vi "frontend3.vi"() -> ()   [LabVIEW 2011]
uses:
  custom_modules/typedefs/preset_control_cluster.ctl
  custom_modules/typedefs/control_cluster.ctl
  custom_modules/typedefs/origin_controls.ctl
  custom_modules/typedefs/single_step_controls.ctl
  custom_modules/typedefs/camera_settings_new.ctl
  custom_modules/typedefs/states_v2.ctl
  <vilib>/event_ctls.llb/eventvkey.ctl
  custom_modules/typedefs/dynamic_data.ctl
  <vilib>/vision/Image Controls.llb/IMAQ Image.ctl
  custom_modules/typedefs/image_type.ctl
  <vilib>/Utility/error.llb/DialogType.ctl
  <userlib>/qcam/QCam.llb/QCam Grab Abort.vi
  stage_modules/Globals.vi
  <vilib>/Utility/file.llb/Read From Spreadsheet File (DBL).vi
  <vilib>/vision/NI_Vision_Development_Module.lvlib
panel:
  in  "test start time":u32
  out "error display":errorcluster
  in  "Tab Control":enum32{"Settings", "Advanced"}(tab)
  in  "Preset controls":T1 {"Presets" items=["10nano.preset", "500sep.preset", "test1.preset", "test2.preset", "test3.preset"]}
  in  "Movement controls":T2={"Nx"=10, "Ny"=10, "X separation"=100, "Y separation"=100}
  in  "File name base":string="<title>_<length>_<sampleID>_<stain>"
  in  "Run test button":bool
  in  "close button":bool
  in  "Origin controls":T3
  in  "Single step controls":T4
  in  "Camera settings":T5={"Gain"=1.0, "Exposure (s)"=0.05, "Preview binning"=2, "Capture binning"=0, "auto expose button"=FALSE} {"Capture binning" items=["1x1", "2x2", "4x4", "8x8"]; "Preview binning" items=["1x1", "2x2", "4x4", "8x8"]; "Exposure (s)" scale=1e-05..1000.0 scale format="%^#_1e"; "Gain" scale=0.451..21.5 scale format="%#_3g"}
  out "Histogram":T6(graph)
  out "Preview":T7(plugin-control)
  in  "camera button":bool
  in  "Image Output directory":path=path "C:/Users/0800706m/Documents/output"
  out "connection indicator":bool
  out "Scan map viewer":T7(plugin-control)
  out "elapsed time":string
  out "estimated remaining":string
  in  "Y offset":dbl
  in  "X offset":dbl
  in  "Minimum no. prediction points":dbl=9.0
  in  "Completion email address":string
  in  "Prediction order":i16=1 min=1 max=2
  in  "Prediction tolerance":dbl=100.0
  in  "Use prediction":bool=TRUE
  in  "Focus offset":dbl
  in  "Focus file path":path
  in  "Focus mode":u16(ring) items=["Autofocus", "Read from file"]
  in  "Well numbering mode":u16(ring)=1 items=["X and Y numbers", "Numbers and letters"]
  in  "No. of wells Y":i32=1
  in  "No. of wells X":i32=1
  in  "Well separation Y":dbl=899.0
  in  "Well separation X":dbl=899.0
  in  "PC connection port":u16(ring)=3 items=["PCI board", "COM 1", "TPL1", "COM3"]
  in  "No. of images in focal stack":i32=1
  in  "Focal stack separation":dbl=1.0
  in  "Preset directory":path=path "C:/Users/0800706m/Documents/GitHub/microscope/presets"
  in  "Focus function":u16(ring)=1 items=["Std dev", "Edges std dev"]
  in  "emergency stop":bool
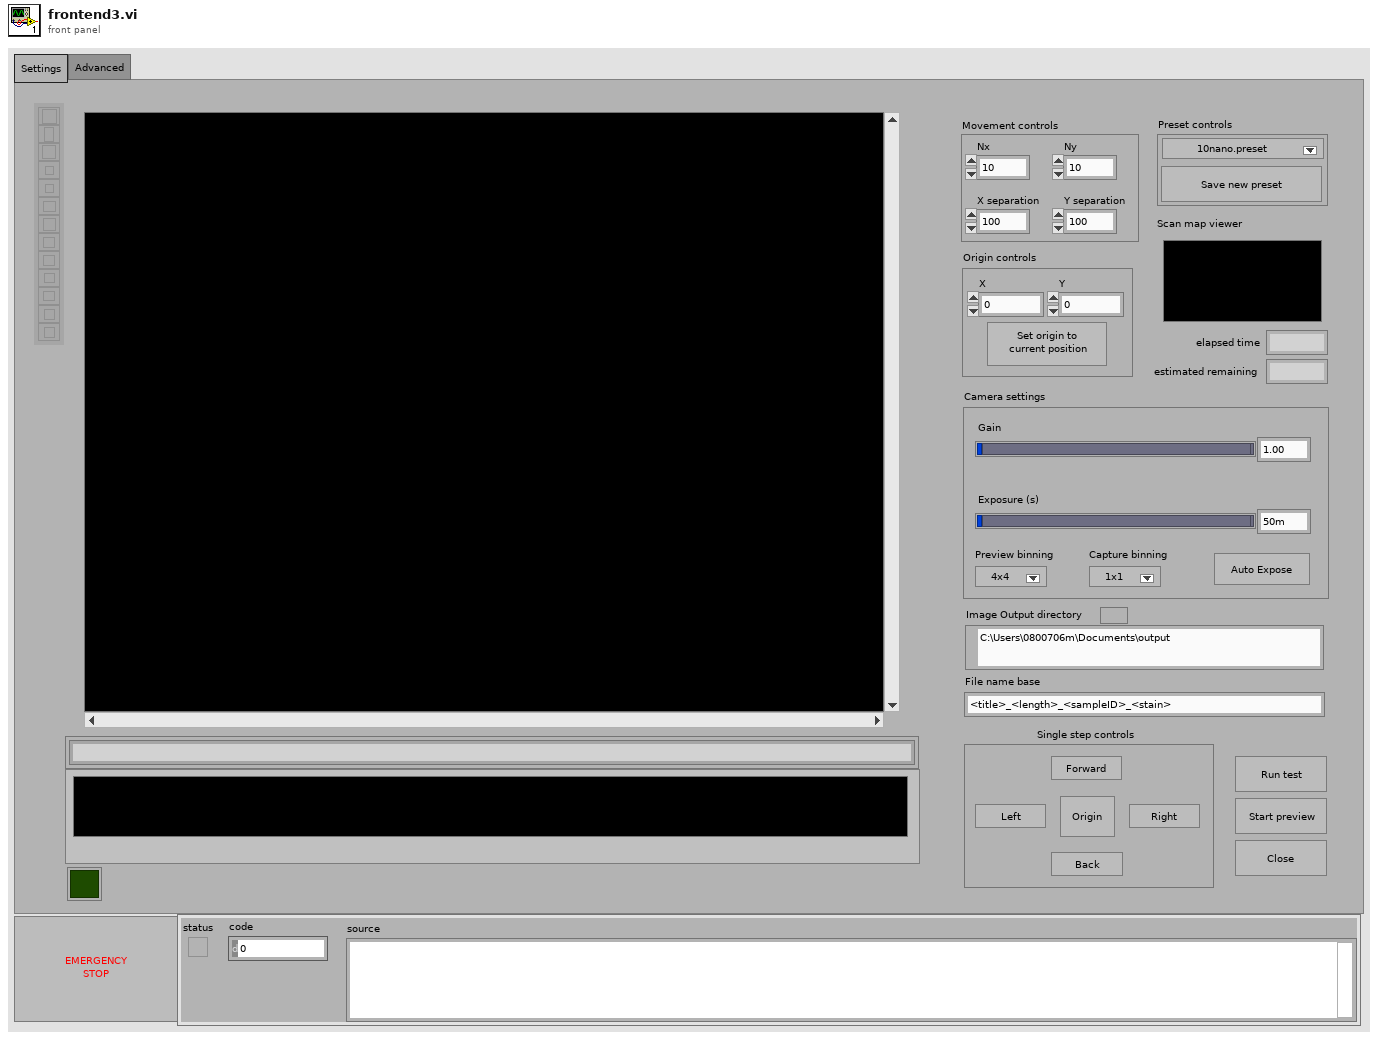
[diagram p1: front panel]
types:
  T1 = typedef "preset_control_cluster.ctl" = cluster{"Presets":u16, "save preset button":bool}
  T2 = typedef "control_cluster.ctl" = cluster{"Nx":i32, "Ny":i32, "X separation":i32, "Y separation":i32}
  T3 = typedef "origin_controls.ctl" = cluster{"X":dbl, "Y":dbl, "set origin button":bool}
  T4 = typedef "single_step_controls.ctl" = cluster{"move to origin button":bool, "Left":bool, "Right":bool, "Back":bool, "Forward":bool}
  T5 = typedef "camera_settings_new.ctl" = cluster{"Gain":dbl, "Exposure (s)":dbl, "Preview binning":u16, "Capture binning":u16, "auto expose button":bool}
  T6 = cluster{"Starting Value":sgl, "Incremental Value":sgl, "Histogram":u32[]}
  T7 = typedef "IMAQ Image.ctl" = refnum<image>
  T8 = typedef "states_v2.ctl" = enum16{"Init", "Preview", "Test init", "Test run", "Test clean", "Close"}
  T9 = typedef "dynamic_data.ctl" = cluster{"PRIORLib.IScanOut":refnum<k7>, "PRIORLib.IStageOut":refnum<k7>, "PRIORLib.IFilterOut":refnum<k7>, "PRIORLib.IZOut":refnum<k7>, "cameraID":u32, "Image Out":T7, "focal map fileref":refnum<file>, "Scan map":T7, "start time":u32, "log fileref":refnum<file>}
  T10 = enum8{"Enabled", "Disabled", "Disabled and Grayed Out"}
  T11 = typedef "image_type.ctl" = enum16{"preview_image", "capture_image"}
  T12 = enum32{"gain", "offset", "exposure", "binning", "horizontal binning", "vertical binning", "readout speed", "trigger type", "lcd filter", "cooler", "exposure red", "exposure blue", "image format", "roi x", "roi y", "roi width", "roi height", "reserved1", "shutter state", "reserved2", "sync-b out", "reserved3", "intensifier gain", "trigger delay", "camera mode", "normalized gain", "normalized intenifier gain DB", "doPostProcessing", "postProcessGainRed", "postProcessGainGreen", "postProcessGainBlue", "postProcessBayerAlgorithm", "postProcessImageFormat", "fan", "blackout mode", "high sensitivity", "Readout Port", "EM Gain", "open delay", "close delay", "clearing mode"}
  T13 = enum16{"open", "replace", "create", "open or create", "replace or create", "replace or create with confirmation"}
  T14 = typedef "Image Type" = u32
  T15 = cluster{"Value":bool, "Value":bool, "Value":bool, "Value":bool, "Value":bool}
  T16 = cluster{"Global Rectangle":i32[], "Contours":cluster{"Contour Type":u32, "ROI Type":u32, "Points":i32[]}[]}
  T17 = typedef "DialogType.ctl" = u16
  T18 = cluster{"stage adjusted":bool, "stage adjusted":bool, "stage adjusted":bool, "stage adjusted":bool, "stage adjusted":bool}
  T19 = cluster{"Movement controls":T2, "Origin controls":T3, "Camera settings":T5, "Image Output directory":path, "File name base":string, "Focal stack separation":dbl, "No. of images in focal stack":i32, "Well separation X":dbl, "Well separation Y":dbl, "No. of wells X":i32, "No. of wells Y":i32, "Well numbering mode":u16, "Focus mode":u16, "Focus file path":path, "Focus offset":dbl, "X offset":dbl, "Y offset":dbl, "Focus function":u16, "Use prediction":bool, "Prediction order":i16, "Prediction tolerance":dbl, "Minimum no. prediction points":dbl}
  T20 = cluster{dbl, dbl, "predicted focal position":dbl}
  T21 = cluster{"Focus position":dbl, "Number of captures":i32}
  T22 = typedef "eventvkey.ctl" = enum16{"ASCII", "Enter", "Return", "Shift", "Ctrl", "Alt", "Cmd", "Opt", "Caps", "NumLock", "Clear", "Break", "Up", "Down", "Left", "Right", "Insert", "Delete", "Home", "End", "PageUp", "PageDown", "Escape", "Help", "Pause", "ScrollLock", "F1", "F2", "F3", "F4", "F5", "F6", "F7", "F8", "F9", "F10", "F11", "F12", "F13", "F14", "F15", "F16", "F17", "F18", "F19", "F20", "F21", "F22", "F23", "F24", "Play", "VolumeUp", "VolumeDown", "Mute", "Two Byte Char"}
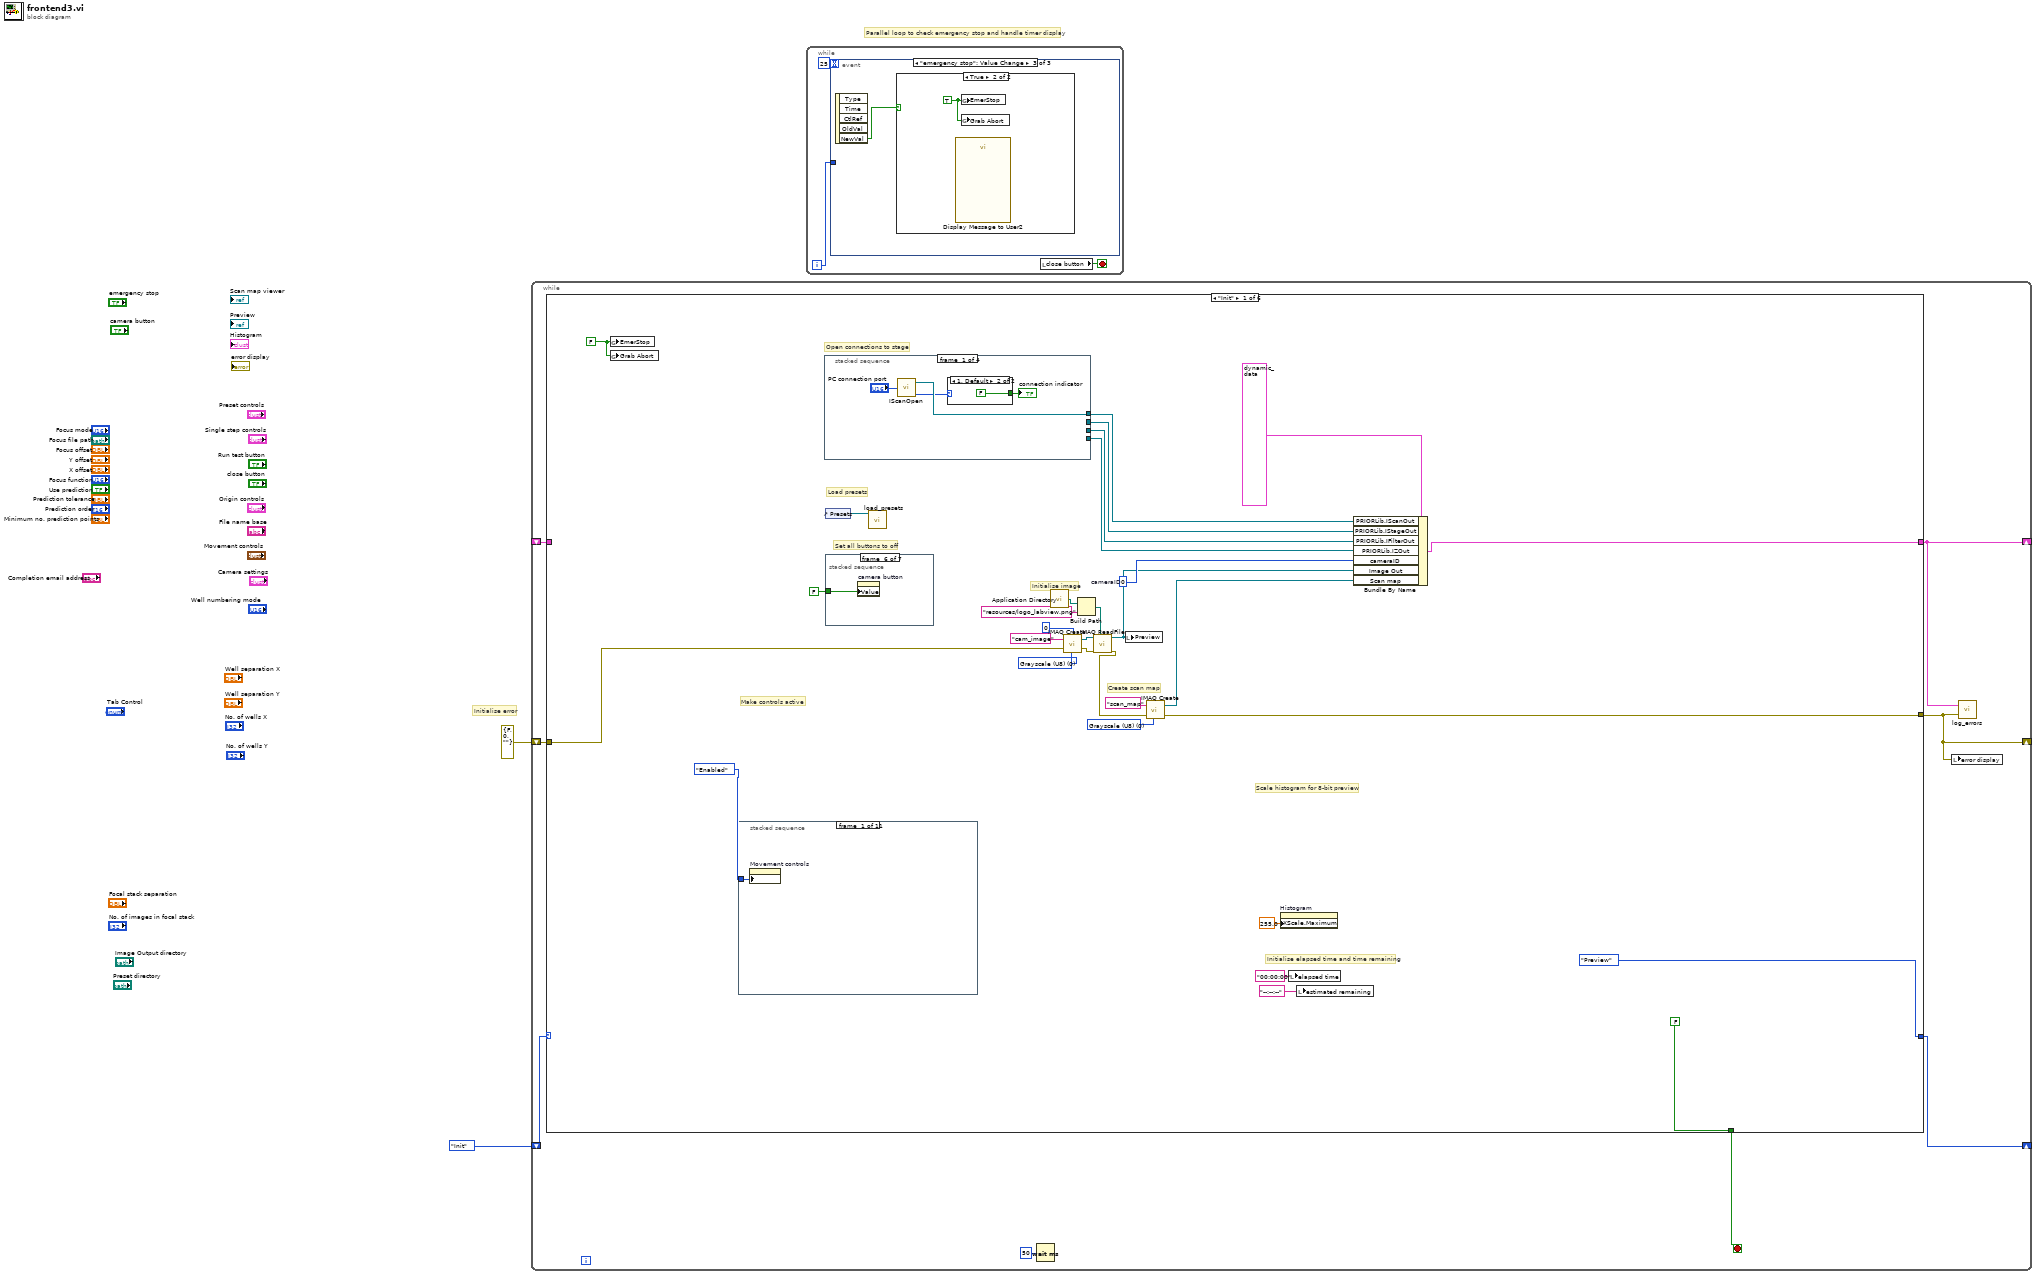
[diagram p0: block diagram]
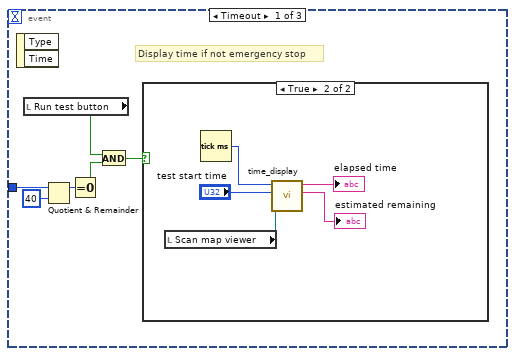
[diagram p2: hidden frame]
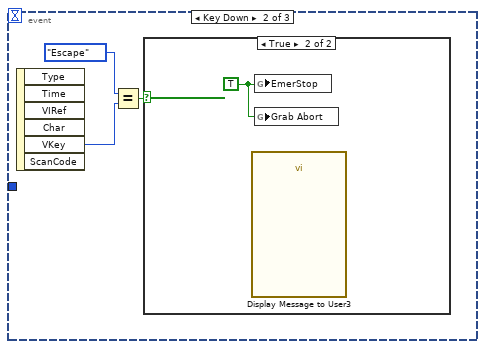
[diagram p4: hidden frame]
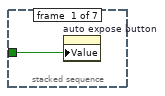
[diagram p7: hidden frame]
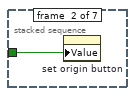
[diagram p8: hidden frame]
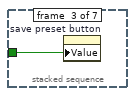
[diagram p9: hidden frame]
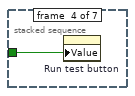
[diagram p10: hidden frame]
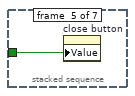
[diagram p11: hidden frame]
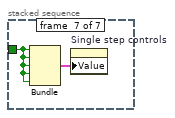
[diagram p12: hidden frame]
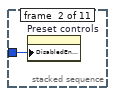
[diagram p13: hidden frame]
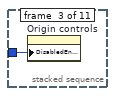
[diagram p14: hidden frame]
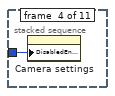
[diagram p15: hidden frame]
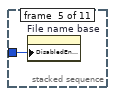
[diagram p16: hidden frame]
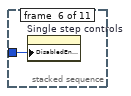
[diagram p17: hidden frame]
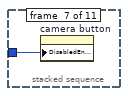
[diagram p18: hidden frame]
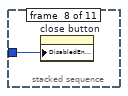
[diagram p19: hidden frame]
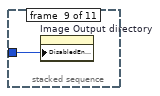
[diagram p20: hidden frame]
diagram:
  # "Initialise error"
  # "Parallel loop to check emergency stop and handle timer display"
  n1 = while {
    shift-right: [w9] -> _
    shift-left: states_v2."Init" -> [w10]
    shift-right: [w4] -> _
    shift-left: _ -> [w6]
    shift-right: [w3] -> _
    shift-left: errorcluster {"status"=FALSE, "code"=0, "source"=""} ("error display") -> [w5]
    stop <- w8 stop-if-true
    n2 = case shown="\"Init\"" w10 {
      tunnel: [states_v2."Preview" w77 w344 states_v2."Test clean" states_v2."Preview" states_v2."Close"] -> w9
      tunnel: [FALSE FALSE FALSE FALSE FALSE TRUE] -> w8
      tunnel: [w21 w75 w347 w428 w782 T9 {"PRIORLib.IScanOut"=refnum, "PRIORLib.IStageOut"=refnum, "PRIORLib.IFilterOut"=refnum, "PRIORLib.IZOut"=refnum, "cameraID"=0, "Image Out"=refnum, "focal map fileref"=refnum, "Scan map"=refnum, "start time"=0, "log fileref"=refnum}] -> w4
      tunnel: w6 -> [_ w74 w366 w428 w790 w824]
      tunnel: [w13 w72 w318 _ w789 w821] -> w3
      tunnel: w5 -> [w12 w73 _ _ w788 w822]
      frame "Init" {
        w11 = FALSE
        w19 = T14 0 items=["Grayscale (U8)", "Grayscale (I16)", "Grayscale (SGL)", "Complex (CSG)", "RGB (U32)", "HSL (U32)", "RGB (U64)", "Grayscale (U16)"] ("Image Type")
        w31 = T14 0 items=["Grayscale (U8)", "Grayscale (I16)", "Grayscale (SGL)", "Complex (CSG)", "RGB (U32)", "HSL (U32)", "RGB (U64)", "Grayscale (U16)"] ("Image Type")
        w30 = u32 0  # cameraID
        # "Initialise elapsed time and time remaining"
        # "Create scan map"
        # "Initialise image"
        # "Scale histogram for 8-bit preview"
        # "Set all buttons to off"
        # "Make controls active"
        # "Open connections to stage"
        # "Load presets"
        n3 = global write "Globals.vi" "EmerStop"(w11) -> ()
        n4 = global write "QCam Grab Abort.vi" "Grab Abort"(w11) -> ()
        n5 = stacked-sequence {
          tunnel: T10."Enabled" ("Disabled") -> [w50 w51 w52 w53 w54 w55 w56 w57 w58 w59 _]
          frame #0 {
            n6 = property on="Movement controls" class="Clust (strict)"("DisabledEnum"=w50) -> ()  [unwired: 2 in, 2 out]
          }
          frame #1 {
            n7 = property on="Preset controls" class="Clust (strict)"("DisabledEnum"=w51) -> ()  [unwired: 2 in, 2 out]
          }
          frame #2 {
            n8 = property on="Origin controls" class="Clust (strict)"("DisabledEnum"=w52) -> ()  [unwired: 2 in, 2 out]
          }
          frame #3 {
            n9 = property on="Camera settings" class="Clust (strict)"("DisabledEnum"=w53) -> ()  [unwired: 2 in, 2 out]
          }
          frame #4 {
            n10 = property on="File name base" class="Str"("DisabledEnum"=w54) -> ()  [unwired: 2 in, 2 out]
          }
          frame #5 {
            n11 = property on="Single step controls" class="Clust (strict)"("DisabledEnum"=w55) -> ()  [unwired: 2 in, 2 out]
          }
          frame #6 {
            n12 = property on="camera button" class="Bool (strict)"("DisabledEnum"=w56) -> ()  [unwired: 2 in, 2 out]
          }
          frame #7 {
            n13 = property on="close button" class="Bool (strict)"("DisabledEnum"=w57) -> ()  [unwired: 2 in, 2 out]
          }
          frame #8 {
            n14 = property on="Image Output directory" class="Path"("DisabledEnum"=w58) -> ()  [unwired: 2 in, 2 out]
          }
          frame #9 {
            n15 = property on="Y offset" class="DigNum (strict)"("DisabledEnum"=w59) -> ()  [unwired: 2 in, 2 out]
            n16 = property on="Focus file path" class="Path"("DisabledEnum"=w59) -> ()  [unwired: 2 in, 2 out]
            n17 = property on="Focus offset" class="DigNum (strict)"("DisabledEnum"=w59) -> ()  [unwired: 2 in, 2 out]
            n18 = property on="X offset" class="DigNum (strict)"("DisabledEnum"=w59) -> ()  [unwired: 2 in, 2 out]
          }
          frame #10 {
            w60 = T10."Disabled and Grayed Out" ("Disabled")
            # "Special case for focus controls"
            n19 = property on="Focus function" class="Ring (strict)"("DisabledEnum"=w60) -> ()  [unwired: 2 in, 2 out]
            n20 = property on="Use prediction" class="Bool (strict)"("DisabledEnum"=w60) -> ()  [unwired: 2 in, 2 out]
            n21 = property on="Prediction order" class="DigNum (strict)"("DisabledEnum"=w60) -> ()  [unwired: 2 in, 2 out]
            n22 = property on="Prediction tolerance" class="DigNum (strict)"("DisabledEnum"=w60) -> ()  [unwired: 2 in, 2 out]
            n23 = property on="Minimum no. prediction points" class="DigNum (strict)"("DisabledEnum"=w60) -> ()  [unwired: 2 in, 2 out]
          }
        }
        n24 = stacked-sequence {
          tunnel: [w64 _ _ _] -> w14
          tunnel: [_ w67 _ _] -> w37
          tunnel: [_ _ w68 _] -> w36
          tunnel: [_ _ _ w69] -> w35
          frame #0 {
            n25 = call "IScanOpen.vi"("Port"="PC connection port") -> ("PRIORLib.IScanOut"=w64:refnum<k7>, "Return"=w63:i32)  [unwired: 1 out]
            n26 = case shown="1, Default" w63 {
              tunnel: [TRUE ("connection indicator") FALSE ("connection indicator")] -> w61
              frame 0 {
              }
              frame 1, Default {
              }
            }
            "connection indicator" <- w61
          }
          frame #1 {
            n27 = call "IStageOpen.vi"() -> ("PRIORLib.IStageOut"=w67:refnum<k7>)  [unwired: 1 in, 1 out]
          }
          frame #2 {
            n28 = call "IFilterOpen.vi"() -> ("PRIORLib.IFilterOut"=w68:refnum<k7>)  [unwired: 1 in, 1 out]
          }
          frame #3 {
            n29 = call "IZOpen.vi"() -> ("PRIORLib.IZOut"=w71:refnum<k7>)  [unwired: 1 in, 1 out]
            n30 = call "IZMaxSpeed.vi"("ZSpeed"=50.0, "PRIORLib.IZIn"=w71) -> ("PRIORLib.IZOut"=w69:refnum<k7>)  [unwired: 1 out]
          }
        }
        n31 = control-ref of="Presets"() -> (w39:refnum<vi>)
        n32 = stacked-sequence {
          tunnel: FALSE ("Value") -> [w42 w43 w44 w45 w46 w47 w48]
          frame #0 {
            n33 = property on="auto expose button" class="Bool (strict)"("Value"=w42) -> ()  [unwired: 2 in, 2 out]
          }
          frame #1 {
            n34 = property on="set origin button" class="Bool (strict)"("Value"=w43) -> ()  [unwired: 2 in, 2 out]
          }
          frame #2 {
            n35 = property on="save preset button" class="Bool (strict)"("Value"=w44) -> ()  [unwired: 2 in, 2 out]
          }
          frame #3 {
            n36 = property on="Run test button" class="Bool (strict)"("Value"=w45) -> ()  [unwired: 2 in, 2 out]
          }
          frame #4 {
            n37 = property on="close button" class="Bool (strict)"("Value"=w46) -> ()  [unwired: 2 in, 2 out]
          }
          frame #5 {
            n38 = property on="camera button" class="Bool (strict)"("Value"=w47) -> ()  [unwired: 2 in, 2 out]
          }
          frame #6 {
            n39 = Bundle("Value"=w48, "Value"=w48, "Value"=w48, "Value"=w48, "Value"=w48) -> (w49:T15)  [unwired: 1 in]
            n40 = property on="Single step controls" class="Clust (strict)"("Value"=w49) -> ()  [unwired: 2 in, 2 out]
          }
        }
        n41 = call "load_presets.vi"("Ring in"=w39) -> ()  [unwired: 10 in, 1 out]
        n42 = call <vilib>:"Application Directory.vi"() -> ("Application Directory"=w25:path)
        n43 = call "IMAQ Create"("Border Size"=0, "Image Name"="cam_image", "Image Type"=w31, "error in (no error)"=w12) -> ("New Image"=w28:T7, "error out"=w27:errorcluster)  [unwired: 1 in]
        n44 = Build Path(base path=w25, name or relative path="resources/logo_labview.png") -> (appended path=w23:path)
        n45 = call "IMAQ ReadFile"("File Path"=w23, "error in (no error)"=w27, "Image"=w28) -> ("error out"=w17:errorcluster, "Image Out"=w26:T7)  [unwired: 4 in, 3 out]
        n46 = local write "Preview"(w26) -> ()
        n47 = call "IMAQ Create"("Image Name"="scan_map", "Image Type"=w19, "error in (no error)"=w17) -> ("New Image"=w18:T7, "error out"=w13:errorcluster)  [unwired: 2 in]
        n48 = property on="Histogram" class="WFGraph (strict)"("XScale.Maximum"=255.0 ("X Scale.Range:Maximum")) -> ()  [unwired: 2 in, 2 out]
        n49 = local write "elapsed time"("00:00:00" ("date/time string")) -> ()
        n50 = local write "estimated remaining"("--:--:--" ("estimated time remaining")) -> ()
        n51 = Bundle By Name(cluster=T9 {"PRIORLib.IScanOut"=refnum, "PRIORLib.IStageOut"=refnum, "PRIORLib.IFilterOut"=refnum, "PRIORLib.IZOut"=refnum, "cameraID"=0, "Image Out"=refnum, "focal map fileref"=refnum, "Scan map"=refnum, "start time"=0, "log fileref"=refnum} ("output cluster"), "PRIORLib.IScanOut"=w14, "PRIORLib.IStageOut"=w37, "PRIORLib.IFilterOut"=w36, "PRIORLib.IZOut"=w35, "cameraID"=w30, "Image Out"=w26, "Scan map"=w18) -> (w21:T9)
      }
      frame "Preview", Default {
        n52 = event shown="[11] \"Single step controls\": Value Change" {
          selector: _ -> [_ _ _ _ _ _ _ _ _ _ _ _ _]
          dyn-events: _ -> [_ _ _ _ _ _ _ _ _ _ _ _ _]
          timeout: 0 -> [_ _ _ _ _ _ _ _ _ _ _ _ _]
          tunnel: [states_v2."Preview" states_v2."Close" states_v2."Preview" states_v2."Preview" states_v2."Preview" states_v2."Preview" states_v2."Preview" w221 states_v2."Preview" states_v2."Preview" states_v2."Preview" states_v2."Preview" states_v2."Preview"] -> w77
          tunnel: w74 -> [w81 w94 w100 w130 w151 w164 w190 w222 w233 w245 w249 w262 w310]
          tunnel: [w81 w94 w98 w130 w151 w167 w190 w222 w233 w245 w249 w262 w310] -> w75
          tunnel: [w80 w93 w96 w129 w148 w162 w185 w219 w225 w234 w247 w260 w312] -> w72
          tunnel: w73 -> [w79 w93 w97 w128 w147 w161 w184 w219 w227 w235 w246 w260 w312]
          event Timeout {
            n53 = event-data() -> ()  [unwired: 1 in, 2 out]
            n54 = Unbundle By Name(w81) -> ("cameraID"=w82:u32)
            n55 = Not Equal To 0?(x=w82) -> (x != 0?=w83:bool)
            n56 = case shown="True" w83 {
              tunnel: w81 -> [_ w90]
              tunnel: [w85 w87] -> w80
              tunnel: w79 -> [w85 w86]
              frame False {
              }
              frame True {
                # "If camera is open, grab and display"
                n57 = Unbundle By Name(w90) -> ("cameraID"=w92:u32, "Image Out"=w91:T7)
                n58 = call <userlib>:"QCAM Grab Acquire.vi"("error in (no error)"=w86, "Image"=w91, "cameraId"=w92) -> ("error out"=w87:errorcluster, "Image Out"=w89:T7)  [unwired: 1 out]
                n59 = call "IMAQ Histograph"("Image"=w89) -> ("Histogram Graph"=w88:T6)  [unwired: 7 in, 3 out]
                n60 = local write "Preview"(w89) -> ()
                n61 = local write "Histogram"(w88) -> ()
              }
            }
          }
          event "close button": Value Change {
            n62 = event-data() -> ()  [unwired: 1 in, 5 out]
          }
          event "camera button": Value Change {
            n63 = event-data() -> ("NewVal"=w101:bool)  [unwired: 1 in, 4 out]
            n64 = case shown="True" w101 {
              tunnel: w100 -> [w107 w120]
              tunnel: [w106 w127] -> w98
              tunnel: [w105 w119] -> w96
              tunnel: w97 -> [w104 w118]
              frame False {
                # "Close camera if button unclicked"
                n65 = flat-sequence {
                  tunnel: w107 -> [w110]
                  tunnel: [w110] -> w103
                  tunnel: [w109] -> w102
                  tunnel: w104 -> [w108]
                  tunnel: w103 -> [w117]
                  tunnel: [w116] -> w106
                  tunnel: [w114] -> w105
                  tunnel: w102 -> [w114]
                  frame #0 {
                    # "Stop capture and camera"
                    n66 = Unbundle By Name(w110) -> ("cameraID"=w111:u32)
                    n67 = call <userlib>:"QCAM Grab Stop.vi"("error in (no error)"=w108, "cameraId"=w111) -> ("error out"=w112:errorcluster, "cameraId Out"=w113:u32)
                    n68 = call <userlib>:"QCAM Close.vi"("error in (no error)"=w112, "cameraId"=w113) -> ("error out"=w109:errorcluster)  [unwired: 1 in]
                  }
                  frame #1 {
                    # "set camera ID to 0"
                    n69 = Bundle By Name(cluster=w117, "cameraID"=u32 0) -> (w116:T9)
                  }
                }
              }
              frame True {
                # "Free original image"
                # "Start camera"
                # "Open camera if button clicked"
                n70 = Unbundle By Name(w120) -> ("Image Out"=w122:T7)
                n71 = call "IMAQ Dispose"("Image"=w122, "error in (no error)"=w118) -> ("error out"=w121:errorcluster)  [unwired: 4 in]
                n72 = local read "Camera settings"() -> (w123:T5)
                n73 = call "start_camera_new.vi"("error in (no error)"=w121, "image type"=image_type."preview_image", "Camera settings"=w123) -> ("error out"=w119:errorcluster, "cameraId out"=w125:u32, "Refnum out"=w124:T7)  [unwired: 5 in, 1 out]
                n74 = Bundle By Name(cluster=w120, "cameraID"=w125, "Image Out"=w124) -> (w127:T9)
              }
            }
          }
          event Value Change {
            # "Handle gain changes"
            n75 = event-data() -> ("NewVal"=w132:dbl)  [unwired: 1 in, 4 out]
            n76 = Unbundle By Name(w130) -> ("cameraID"=w131:u32)
            n77 = Not Equal To 0?(x=w131) -> (x != 0?=w134:bool)
            n78 = case shown="True" w134 {
              tunnel: w132 -> [_ w139]
              tunnel: w131 -> [_ w138]
              tunnel: [w135 w137] -> w129
              tunnel: w128 -> [w135 w136]
              frame False {
              }
              frame True {
                n79 = Divide(x=w139, y=0.451) -> (x/y=w143:dbl)
                n80 = Logarithm Base X(1:1.000944118 ("x"), 2:w143) -> (0:w141:dbl)
                n81 = To Long Integer(number=w141) -> (32bit integer=w140:i32)
                n82 = call <userlib>:"QCAM SetParam.vi"("error in (no error)"=w136, "value"=w140, "parameter key"=T12."gain", "cameraId"=w138) -> ("error out"=w137:errorcluster)  [unwired: 1 out]
              }
            }
          }
          event Value Change {
            # "Handle exposure changes"
            n83 = event-data() -> ("NewVal"=w150:dbl)  [unwired: 1 in, 4 out]
            n84 = Unbundle By Name(w151) -> ("cameraID"=w149:u32)
            n85 = Not Equal To 0?(x=w149) -> (x != 0?=w152:bool)
            n86 = case shown="False" w152 {
              tunnel: w150 -> [_ w157]
              tunnel: w149 -> [_ w156]
              tunnel: [w153 w155] -> w148
              tunnel: w147 -> [w153 w154]
              frame False {
              }
              frame True {
                n87 = Multiply(x=w157, y=1000000.0 ("x")) -> (x*y=w160:dbl)
                n88 = call <userlib>:"QCAM SetParam.vi"("error in (no error)"=w154, "value"=w160, "parameter key"=T12."exposure", "cameraId"=w156) -> ("error out"=w155:errorcluster)  [unwired: 1 out]
              }
            }
          }
          event Value Change {
            # "Handle binning changes"
            n89 = event-data() -> ()  [unwired: 1 in, 5 out]
            n90 = Unbundle By Name(w164) -> ("cameraID"=w166:u32)
            n91 = Not Equal To 0?(x=w166) -> (x != 0?=w165:bool)
            n92 = case shown="True" w165 {
              tunnel: w164 -> [w169 w171]
              tunnel: [w169 w183] -> w167
              tunnel: [w168 w182] -> w162
              tunnel: w161 -> [w168 w170]
              frame False {
              }
              frame True {
                # "start camera with new binning"
                # "stop camera and free image"
                n93 = Unbundle By Name(w171) -> ("cameraID"=w179:u32, "Image Out"=w180:T7)
                n94 = call <userlib>:"QCAM Grab Stop.vi"("error in (no error)"=w170, "cameraId"=w179) -> ("error out"=w178:errorcluster, "cameraId Out"=w177:u32)
                n95 = call <userlib>:"QCAM Close.vi"("error in (no error)"=w178, "cameraId"=w177) -> ("error out"=w181:errorcluster)  [unwired: 1 in]
                n96 = call "IMAQ Dispose"("Image"=w180, "error in (no error)"=w181) -> ("error out"=w172:errorcluster)  [unwired: 4 in]
                n97 = local read "Camera settings"() -> (w173:T5)
                n98 = call "start_camera_new.vi"("error in (no error)"=w172, "image type"=image_type."preview_image", "Camera settings"=w173) -> ("error out"=w182:errorcluster, "cameraId out"=w175:u32, "Refnum out"=w174:T7)  [unwired: 5 in, 1 out]
                n99 = Bundle By Name(cluster=w171, "cameraID"=w175, "Image Out"=w174) -> (w183:T9)
              }
            }
          }
          event Value Change {
            # "Auto expose from ROI or full image if there is no ROI"
            # "Update exposure slider"
            n100 = event-data() -> ()  [unwired: 1 in, 5 out]
            n101 = Unbundle By Name(w190) -> ("cameraID"=w193:u32, "Image Out"=w192:T7)
            n102 = property on="Preview" class="ImageControl"() -> ("ROI"=w194:T16)  [unwired: 2 in, 2 out]
            n103 = Unbundle(w194) -> ("Global Rectangle"=w197:i32[])  [unwired: 1 out]
            n104 = Array Size(array=w197) -> (size(s)=w198:i32)
            n105 = Not Equal To 0?(x=w198) -> (x != 0?=w199:bool)
            n106 = case shown="True" w199 {
              tunnel: w197 -> [_ w216]
              tunnel: [w208 w215] -> w200
              tunnel: [w208 w214] -> w201
              tunnel: [w209 w213] -> w202
              tunnel: [w210 w212] -> w203
              tunnel: w192 -> [w207 _]
              tunnel: [w206 w211] -> w189
              tunnel: w184 -> [w205 w211]
              frame False {
                w208 = 0
                n107 = call "IMAQ GetImageSize"("Image"=w207, "error in (no error)"=w205) -> ("Y Resolution"=w210:i32, "X Resolution"=w209:i32, "error out"=w206:errorcluster)  [unwired: 2 in]
              }
              frame True {
                n108 = Index Array(array=w216) -> (element #1=w215:i32, element #2=w214:i32, element #3=w218:i32, element #4=w217:i32)  [unwired: 4 in]
                n109 = Subtract(x=w218, y=w215) -> (x-y=w213:i32)
                n110 = Subtract(x=w217, y=w214) -> (x-y=w212:i32)
              }
            }
            n111 = call <userlib>:"QCAM AutoExpose.vi"("xOrig"=w200, "cameraId"=w193, "yOrig"=w201, "width"=w202, "error in (no error)"=w189, "height"=w203) -> ("cameraId out"=w196:u32, "error out"=w195:errorcluster)  [unwired: 1 in]
            n112 = call <userlib>:"QCAM GetParam.vi"("cameraId in"=w196, "parameter key"=T12."exposure", "error in (no error)"=w195) -> ("value out"=w186:u32, "error out"=w185:errorcluster)  [unwired: 3 out]
            n113 = Divide(x=w186, y=u32 1000000 ("x")) -> (x/y=w188:dbl)
            n114 = property on="Exposure (s)" class="Slide (strict)"("Value"=w188) -> ()  [unwired: 2 in, 2 out]
          }
          event "Run test button": Value Change {
            # "Go to test mode"
            n115 = event-data() -> ("NewVal"=w220:bool)  [unwired: 1 in, 4 out]
            n116 = case shown="True" w220 {
              tunnel: [states_v2."Preview" states_v2."Test init"] -> w221
              frame False {
              }
              frame True {
              }
            }
          }
          event Value Change {
            # "Restore button"
            # "Change origin if button has been pressed"
            # "Get current position from stage and use as origin"
            n117 = event-data() -> ()  [unwired: 1 in, 5 out]
            n118 = Unbundle By Name(w233) -> ("PRIORLib.IStageOut"=w228:refnum<k7>)
            n119 = invoke class="IStage" method="GetPosition"(reference=w228, error in=w227) -> (error out=w226:errorcluster, "XPos"=w231:dbl, "YPos"=w230:dbl)  [unwired: 3 in, 2 out]
            n120 = property on="X" class="DigNum (strict)"("Value"=w231) -> ()  [unwired: 2 in, 2 out]
            n121 = property on="Y" class="DigNum (strict)"("Value"=w230) -> ()  [unwired: 2 in, 2 out]
            n122 = property on="set origin button" class="Bool (strict)"(error in=w226, "Value"=FALSE ("set origin button")) -> (error out=w225:errorcluster)  [unwired: 1 in, 1 out]
          }
          event Value Change {
            w242 = T17 0 items=["no dialog", "OK message", "continue or stop message", "OK message + warnings", "continue/stop + warnings"] ("type of dialog (OK msg:1)")
            # "Restore button"
            # "Reload preset list"
            # "Save controls as XML preset and ignore errors"
            # "Save current settings as preset"
            n123 = event-data() -> ()  [unwired: 1 in, 5 out]
            n124 = local read "Movement controls"() -> (w243:T2)
            n125 = Flatten To XML(anything=w243) -> (xml string=w240:string)
            n126 = Write to Text File(text=w240, error in=w235) -> (error out=w241:errorcluster)  [unwired: 2 in, 2 out]
            n127 = call <vilib>:"Simple Error Handler.vi"("type of dialog (OK msg:1)"=w242, "error in (no error)"=w241) -> ("error out"=w237:errorcluster)  [unwired: 3 in, 4 out]
            n128 = control-ref of="Presets"() -> (w239:refnum<vi>)
            n129 = call "load_presets.vi"("error in"=w237, "Ring in"=w239) -> ("error out"=w236:errorcluster)  [unwired: 9 in]
            n130 = property on="save preset button" class="Bool (strict)"(error in=w236, "Value"=FALSE) -> (error out=w234:errorcluster)  [unwired: 1 in, 1 out]
          }
          event Value Change {
            # "Get currently selected preset and load into controls"
            # "List \".preset\" files in preset folder"
            n131 = event-data() -> ("NewVal"=w250:u16)  [unwired: 1 in, 4 out]
            n132 = local read "Preset directory"() -> (w259:path)
            n133 = List Folder(path=w259, pattern="*.preset") -> (filenames=w253:string[])  [unwired: 2 in, 3 out]
            n134 = Index Array(array=w253, index=w250) -> (element=w252:string)
            n135 = Build Path(base path=w259, name or relative path=w252) -> (appended path=w256:path)
            n136 = Read from Text File(file (use dialog)=w256, error in=w246) -> (text=w258:string, error out=w257:errorcluster)  [unwired: 2 in, 2 out]
            n137 = Unflatten From XML(xml string=w258, type=T2 {"Nx"=0, "Ny"=0, "X separation"=0, "Y separation"=0} ("controls"), error in (no error)=w257) -> (value=w251:T2, error out=w247:errorcluster)
            n138 = local write "Movement controls"(w251) -> ()
          }
          event Value Change {
            # "Cycle through buttons and execute the one that has been pressed"
            # "Move stage by 1 step.\nSize of step is determined by movement controls"
            n139 = event-data() -> ()  [unwired: 1 in, 5 out]
            n140 = Unbundle By Name(w262) -> ("PRIORLib.IScanOut"=w261:refnum<k7>)
            n141 = local read "Movement controls"() -> (w266:T2)
            n142 = local read "Single step controls"() -> (w263:T4)
            n143 = Unbundle By Name(w266) -> ("X separation"=w264:i32, "Y separation"=w265:i32)
            n144 = stacked-sequence {
              tunnel: w261 -> [w270 w276 w284 w291 w299 _]
              tunnel: w263 -> [w268 w279 w287 w294 w302 _]
              tunnel: w265 -> [_ _ _ w292 w300 _]
              tunnel: w264 -> [_ w277 w285 _ _ _]
              frame #0 {
                n145 = Unbundle By Name(w268) -> ("move to origin button"=w269:bool)
                n146 = case shown="True" w269 {
                  tunnel: w270 -> [_ w271]
                  frame False {
                  }
                  frame True {
                    n147 = local read "Origin controls"() -> (w275:T3)
                    n148 = Unbundle By Name(w275) -> ("X"=w273:dbl, "Y"=w272:dbl)
                    n149 = call "IScanMoveXYZAbs.vi"("PRIORLib.IScanIn"=w271, "XPos"=w273, "YPos"=w272, "ZPos"=0.0) -> ()  [unwired: 1 in, 3 out]
                  }
                }
              }
              frame #1 {
                n150 = Unbundle By Name(w279) -> ("Left"=w278:bool)
                n151 = case shown="True" w278 {
                  tunnel: w277 -> [_ w283]
                  tunnel: w276 -> [_ w280]
                  frame False {
                  }
                  frame True {
                    w281 = 0.0 ("ZPos")
                    n152 = Negate(x=w283) -> (-x=w282:i32)
                    n153 = call "IScanMoveXYZ.vi"("ZPos"=w281, "YPos"=w281, "XPos"=w282, "PRIORLib.IScanIn"=w280) -> ()  [unwired: 3 out]
                  }
                }
              }
              frame #2 {
                n154 = Unbundle By Name(w287) -> ("Right"=w286:bool)
                n155 = case shown="True" w286 {
                  tunnel: w285 -> [_ w289]
                  tunnel: w284 -> [_ w288]
                  frame False {
                  }
                  frame True {
                    w290 = 0.0 ("ZPos")
                    n156 = call "IScanMoveXYZ.vi"("ZPos"=w290, "YPos"=w290, "XPos"=w289, "PRIORLib.IScanIn"=w288) -> ()  [unwired: 3 out]
                  }
                }
              }
              frame #3 {
                n157 = Unbundle By Name(w294) -> ("Back"=w293:bool)
                n158 = case shown="True" w293 {
                  tunnel: w292 -> [_ w298]
                  tunnel: w291 -> [_ w295]
                  frame False {
                  }
                  frame True {
                    w296 = 0.0 ("ZPos")
                    n159 = Negate(x=w298) -> (-x=w297:i32)
                    n160 = call "IScanMoveXYZ.vi"("ZPos"=w296, "YPos"=w297, "XPos"=w296, "PRIORLib.IScanIn"=w295) -> ()  [unwired: 3 out]
                  }
                }
              }
              frame #4 {
                n161 = Unbundle By Name(w302) -> ("Forward"=w301:bool)
                n162 = case shown="True" w301 {
                  tunnel: w300 -> [_ w305]
                  tunnel: w299 -> [_ w303]
                  frame False {
                  }
                  frame True {
                    w304 = 0.0 ("ZPos")
                    n163 = call "IScanMoveXYZ.vi"("ZPos"=w304, "YPos"=w305, "XPos"=w304, "PRIORLib.IScanIn"=w303) -> ()  [unwired: 3 out]
                  }
                }
              }
              frame #5 {
                w307 = FALSE ("stage adjusted")
                # "restore all buttons"
                n164 = Bundle("stage adjusted"=w307, "stage adjusted"=w307, "stage adjusted"=w307, "stage adjusted"=w307, "stage adjusted"=w307) -> (w306:T18)  [unwired: 1 in]
                n165 = local write "Single step controls"(w306) -> ()
              }
            }
          }
          event "Focus mode": Value Change {
            # "Activate or deactive focus options when switching focus modes"
            n166 = event-data() -> ("NewVal"=w313:u16)  [unwired: 1 in, 4 out]
            n167 = case shown="1" w313 {
              tunnel: [T10."Disabled and Grayed Out" ("Disabled") T10."Enabled" ("Disabled")] -> w309
              tunnel: [T10."Enabled" ("Disabled") T10."Disabled and Grayed Out" ("Disabled")] -> w308
              frame 0, Default {
              }
              frame 1 {
              }
            }
            n168 = property on="Y offset" class="DigNum (strict)"("DisabledEnum"=w309) -> ()  [unwired: 2 in, 2 out]
            n169 = property on="Focus file path" class="Path"("DisabledEnum"=w309) -> ()  [unwired: 2 in, 2 out]
            n170 = property on="Focus offset" class="DigNum (strict)"("DisabledEnum"=w309) -> ()  [unwired: 2 in, 2 out]
            n171 = property on="X offset" class="DigNum (strict)"("DisabledEnum"=w309) -> ()  [unwired: 2 in, 2 out]
            n172 = property on="Focus function" class="Ring (strict)"("DisabledEnum"=w308) -> ()  [unwired: 2 in, 2 out]
            n173 = property on="Use prediction" class="Bool (strict)"("DisabledEnum"=w308) -> ()  [unwired: 2 in, 2 out]
            n174 = property on="Prediction order" class="DigNum (strict)"("DisabledEnum"=w308) -> ()  [unwired: 2 in, 2 out]
            n175 = property on="Prediction tolerance" class="DigNum (strict)"("DisabledEnum"=w308) -> ()  [unwired: 2 in, 2 out]
            n176 = property on="Minimum no. prediction points" class="DigNum (strict)"("DisabledEnum"=w308) -> ()  [unwired: 2 in, 2 out]
          }
        }
      }
      frame "Test init" {
        w360 = T17 0 items=["no dialog", "OK message", "continue or stop message", "OK message + warnings", "continue/stop + warnings"] ("type of dialog (OK msg:1)")
        # "Begin logfile"
        # "Initialise scan map"
        # "Rescale histogram for 12-bit pixels"
        # "If an error occured, go straight to cleanup. Otherwise run the test."
        # "Stop camera if it's still running"
        # "Make controls inactive"
        # "check if file name is blank"
        n177 = local read "File name base"() -> (w386:string)
        n178 = Equal?(x=w386, y="<title>_<length>_<sampleID>_<stain>") -> (x = y?=w387:bool)
        n179 = case shown="True" w387 {
          tunnel: [errorcluster {"status"=FALSE, "code"=0, "source"=""} ("error out") w425] -> w383
          frame False {
          }
          frame True {
            n180 = call "No file name base given!"() -> ("File name base"=w426:string, "error out"=w425:errorcluster)  [unwired: 17 in, 1 out]
            n181 = local write "File name base"(w426) -> ()
          }
        }
        n182 = local read "camera button"() -> (w384:bool)
        n183 = case shown="True" w384 {
          tunnel: [errorcluster {"status"=FALSE, "code"=0, "source"=""} ("error out") w409] -> w380
          tunnel: w383 -> [_ w412]
          tunnel: w366 -> [_ w406]
          frame False {
          }
          frame True {
            n184 = Unbundle By Name(w406) -> ("Image Out"=w408:T7, "cameraID"=w411:u32)
            n185 = call <userlib>:"QCAM Grab Stop.vi"("error in (no error)"=w412, "cameraId"=w411) -> ("error out"=w413:errorcluster, "cameraId Out"=w414:u32)
            n186 = local write "camera button"(FALSE ("camera button")) -> ()
            n187 = call <userlib>:"QCAM Close.vi"("error in (no error)"=w413, "cameraId"=w414) -> ("error out"=w410:errorcluster)  [unwired: 1 in]
            n188 = call "IMAQ Dispose"("Image"=w408, "error in (no error)"=w410) -> ("error out"=w409:errorcluster)  [unwired: 4 in]
          }
        }
        n189 = stacked-sequence {
          tunnel: T10."Disabled and Grayed Out" ("Disabled") -> [w415 w416 w417 w418 w419 w420 w421 w422 w423]
          frame #0 {
            n190 = property on="Movement controls" class="Clust (strict)"("DisabledEnum"=w415) -> ()  [unwired: 2 in, 2 out]
          }
          frame #1 {
            n191 = property on="Preset controls" class="Clust (strict)"("DisabledEnum"=w416) -> ()  [unwired: 2 in, 2 out]
          }
          frame #2 {
            n192 = property on="Camera settings" class="Clust (strict)"("DisabledEnum"=w417) -> ()  [unwired: 2 in, 2 out]
          }
          frame #3 {
            n193 = property on="File name base" class="Str"("DisabledEnum"=w418) -> ()  [unwired: 2 in, 2 out]
          }
          frame #4 {
            n194 = property on="Image Output directory" class="Path"("DisabledEnum"=w419) -> ()  [unwired: 2 in, 2 out]
          }
          frame #5 {
            n195 = property on="Origin controls" class="Clust (strict)"("DisabledEnum"=w420) -> ()  [unwired: 2 in, 2 out]
          }
          frame #6 {
            n196 = property on="Single step controls" class="Clust (strict)"("DisabledEnum"=w421) -> ()  [unwired: 2 in, 2 out]
          }
          frame #7 {
            n197 = property on="camera button" class="Bool (strict)"("DisabledEnum"=w422) -> ()  [unwired: 2 in, 2 out]
          }
          frame #8 {
            n198 = property on="close button" class="Bool (strict)"("DisabledEnum"=w423) -> ()  [unwired: 2 in, 2 out]
          }
        }
        n199 = property on="Histogram" class="WFGraph (strict)"("XScale.Maximum"=4096.0 ("X Scale.Range:Maximum")) -> ()  [unwired: 2 in, 2 out]
        n200 = local read "Focus mode"() -> (w358:u16)
        n201 = local read "Image Output directory"() -> (w359:path)
        n202 = Create Folder(path (use dialog)=w359) -> (created path=w350:path, error out=w357:errorcluster)  [unwired: 2 in, 1 out]
        n203 = case shown="0, Default" w358 {
          tunnel: w380 -> [w400 w404]
          tunnel: [w391 w404] -> w345
          tunnel: w350 -> [w396 _]
          tunnel: [w392 _] -> w346
          frame 0, Default {
            n204 = local read "File name base"() -> (w399:string)
            n205 = Concatenate Strings(w399, "_focal_map.csv" ("name or relative path")) -> (w397:string)
            n206 = Build Path(base path=w396, name or relative path=w397) -> (appended path=w401:path)
            n207 = Open/Create/Replace File(file path (use dialog)=w401, error in=w400, operation (0:open)=T13."replace or create", access (0:read/write)=enum16{"read/write", "read-only", "write-only"}."write-only") -> (refnum out=w394:refnum<file>, error out=w393:errorcluster)  [unwired: 2 in, 1 out]
            n208 = call "CSV header"() -> ("Result"=w395:string)  [unwired: 14 in, 1 out]
            n209 = Write to Text File(file (use dialog)=w394, text=w395, error in=w393) -> (refnum out=w392:refnum<file>, error out=w391:errorcluster)  [unwired: 1 in, 1 out]
          }
          frame 1 {
          }
        }
        n210 = call <vilib>:"Simple Error Handler.vi"("type of dialog (OK msg:1)"=w360, "error in (no error)"=w357) -> ()  [unwired: 3 in, 5 out]
        n211 = local read "File name base"() -> (w354:string)
        n212 = local read "Movement controls"() -> (w373:T2)
        n213 = local read "No. of wells X"() -> (w370:i32)
        n214 = local read "No. of wells Y"() -> (w368:i32)
        n215 = Concatenate Strings(w354, ".log" ("name or relative path")) -> (w356:string)
        n216 = Build Path(base path=w350, name or relative path=w356) -> (appended path=w351:path)
        n217 = Unbundle By Name(w373) -> ("Nx"=w371:i32, "Ny"=w372:i32)
        n218 = Increment(x=w371) -> (x+1=w369:i32)
        n219 = Increment(x=w372) -> (x+1=w367:i32)
        n220 = Open/Create/Replace File(file path (use dialog)=w351, operation (0:open)=T13."replace or create", access (0:read/write)=enum16{"read/write", "read-only", "write-only"}."write-only") -> (refnum out=w348:refnum<file>)  [unwired: 3 in, 2 out]
        n221 = Multiply(x=w370, y=w369) -> (x*y=w364:i32)
        n222 = Multiply(x=w368, y=w367) -> (x*y=w363:i32)
        n223 = Decrement(x=w364) -> (x-1=w361:i32)
        n224 = Decrement(x=w363) -> (x-1=w362:i32)
        n225 = Unbundle By Name(w366) -> ("Scan map"=w374:T7)
        n226 = call "IMAQ SetImageSize"("error in (no error)"=w345, "Y Resolution"=w362, "X Resolution"=w361, "Image"=w374) -> ("error out"=w375:errorcluster, "Image Out"=w377:T7)  [unwired: 1 in]
        n227 = call "IMAQ FillImage"("error in (no error)"=w375, "Pixel Value (U8, U16, I16, Float)"=i8 0, "Image"=w377) -> ("error out"=w319:errorcluster, "Image Out"=w349:T7)  [unwired: 7 in]
        n228 = Unbundle By Name(w319) -> ("status"=w381:bool)
        n229 = Select(t=states_v2."Test clean", s=w381, f=states_v2."Test run") -> (s? t:f=w344:T8)
        n230 = local write "Scan map viewer"(w349) -> ()
        n231 = Bundle By Name(cluster=w366, "cameraID"=u32 0, "focal map fileref"=w346, "log fileref"=w348, "Scan map"=w349) -> (w347:T9)
        n232 = Tick Count (ms)() -> (millisecond timer value=w365:u32)
        n233 = local write "test start time"(w365) -> ()
        n234 = local read "Minimum no. prediction points"() -> (w342:dbl)
        n235 = local read "No. of images in focal stack"() -> (w327:i32)
        n236 = local read "Image Output directory"() -> (w324:path)
        n237 = local read "Well numbering mode"() -> (w332:u16)
        n238 = local read "Focal stack separation"() -> (w326:dbl)
        n239 = local read "Prediction tolerance"() -> (w341:dbl)
        n240 = local read "Movement controls"() -> (w321:T2)
        n241 = local read "Well separation X"() -> (w328:dbl)
        n242 = local read "Well separation Y"() -> (w329:dbl)
        n243 = local read "Camera settings"() -> (w323:T5)
        n244 = local read "Prediction order"() -> (w340:i16)
        n245 = local read "Origin controls"() -> (w322:T3)
        n246 = local read "Focus function"() -> (w338:u16)
        n247 = local read "File name base"() -> (w325:string)
        n248 = local read "Focus file path"() -> (w334:path)
        n249 = local read "Use prediction"() -> (w339:bool)
        n250 = local read "No. of wells X"() -> (w330:i32)
        n251 = local read "No. of wells Y"() -> (w331:i32)
        n252 = local read "Focus mode"() -> (w333:u16)
        n253 = local read "Focus offset"() -> (w335:dbl)
        n254 = local read "X offset"() -> (w336:dbl)
        n255 = local read "Y offset"() -> (w337:dbl)
        n256 = Bundle("Movement controls"=w321, "Origin controls"=w322, "Camera settings"=w323, "Image Output directory"=w324, "File name base"=w325, "Focal stack separation"=w326, "No. of images in focal stack"=w327, "Well separation X"=w328, "Well separation Y"=w329, "No. of wells X"=w330, "No. of wells Y"=w331, "Well numbering mode"=w332, "Focus mode"=w333, "Focus file path"=w334, "Focus offset"=w335, "X offset"=w336, "Y offset"=w337, "Focus function"=w338, "Use prediction"=w339, "Prediction order"=w340, "Prediction tolerance"=w341, "Minimum no. prediction points"=w342) -> (w343:T19)  [unwired: 1 in]
        n257 = Unbundle By Name(w347) -> ("log fileref"=w320:refnum<file>)
        n258 = call "start_log_file.vi"("error in (no error)"=w319, "Cluster"=w343, "log file"=w320) -> ("error out"=w318:errorcluster)
      }
      frame "Test run" {
        n259 = local read "Focus mode"() -> (w427:u16)
        n260 = case shown="1" w427 {
          tunnel: w428 -> [w431 w672]
          frame 0, Default {
            n261 = local read "No. of wells Y"() -> (w432:i32)
            n262 = for {
              N: w432 -> [_]
              tunnel: w431 -> [w433]
              i -> [w434]
              # "Wj"
              n263 = local read "No. of wells X"() -> (w435:i32)
              n264 = for {
                N: w435 -> [w436]
                tunnel: w434 -> [w438]
                tunnel: w433 -> [w437]
                i -> [w439]
                # "Wi"
                n265 = local read "Movement controls"() -> (w441:T2)
                n266 = Unbundle By Name(w441) -> ("Ny"=w440:i32)
                n267 = for {
                  N: w440 -> [_]
                  tunnel: w439 -> [w445]
                  tunnel: w438 -> [w444]
                  tunnel: w437 -> [w443]
                  tunnel: w436 -> [w442]
                  i -> [w446]
                  # "Nj"
                  n268 = local read "Movement controls"() -> (w448:T2)
                  n269 = Unbundle By Name(w448) -> ("Nx"=w447:i32)
                  n270 = for {
                    N: w447 -> [w450]
                    tunnel: w446 -> [w457]
                    tunnel: w445 -> [w455]
                    tunnel: w444 -> [w456]
                    tunnel: w443 -> [w454]
                    tunnel: w442 -> [w449]
                    i -> [w451]
                    # "If test is aborted, go through the rest of the loop iterations, but do nothing"
                    # "Ni"
                    n271 = local read "Run test button"() -> (w453:bool)
                    n272 = Not(x=w453) -> (.not. x?=w452:bool)
                    n273 = case shown="False" w452 {
                      tunnel: w457 -> [w464 _]
                      tunnel: w451 -> [w463 _]
                      tunnel: w456 -> [w462 _]
                      tunnel: w455 -> [w461 _]
                      tunnel: w454 -> [w460 _]
                      tunnel: w450 -> [w459 _]
                      tunnel: w449 -> [w458 _]
                      frame False {
                        # "Nx"
                        # "Wnx"
                        # "true Ni,Wi"
                        # "focus position used, no. captures"
                        # "x,y,z"
                        n274 = stacked-sequence {
                          seq-local: [w481 _ _ _ _ _ _ _] -> [_ w536 _ _ _ _ _ w668]
                          seq-local: [_ _ w543 _ _ _ _ _] -> [_ _ _ _ _ _ w643 w663]
                          seq-local: [w475 _ _ _ _ _ _ _] -> [_ _ _ _ w570 w628 _ w657]
                          tunnel: w464 -> [w472 _ _ _ w589 w629 _ w664]
                          tunnel: w463 -> [w473 _ _ _ _ _ _ _]
                          tunnel: w462 -> [w474 _ _ _ w587 w630 _ w665]
                          tunnel: w461 -> [w480 _ _ _ _ _ _ _]
                          tunnel: w460 -> [w470 w538 w544 w568 w576 w634 w646 w660]
                          tunnel: w459 -> [w478 _ _ _ _ _ _ _]
                          tunnel: w458 -> [w479 _ _ _ _ _ _ _]
                          frame #0 {
                            # "Predict focus position, and use for movement"
                            # "Start new entry in logfile"
                            # "Meander through wells and images within wells"
                            # "calculate Y"
                            # "calculate X"
                            n275 = call "meander.vi"("Wnx"=w479, "Wi"=w480, "Wj"=w474, "Nx"=w478, "Ni"=w473, "Nj"=w472) -> ("Wi new"=w476:i32, "Ni new"=w477:i32)  [unwired: 12 in]
                            n276 = Bundle("Wi new"=w476, "Ni new"=w477) -> (w475:cluster{"Wi new":i32, "Ni new":i32})  [unwired: 1 in]
                            n277 = local read "Movement controls"() -> (w502:T2)
                            n278 = local read "Well separation X"() -> (w498:dbl)
                            n279 = local read "Well separation Y"() -> (w499:dbl)
                            n280 = Unbundle By Name(w502) -> ("X separation"=w500:i32)
                            n281 = Unbundle By Name(w502) -> ("Y separation"=w501:i32)
                            n282 = local read "Origin controls"() -> (w493:T3)
                            n283 = Multiply(x=w498, y=w476) -> (x*y=w497:dbl)
                            n284 = Multiply(x=w500, y=w477) -> (x*y=w496:i32)
                            n285 = Multiply(x=w499, y=w474) -> (x*y=w494:dbl)
                            n286 = Multiply(x=w501, y=w472) -> (x*y=w495:i32)
                            n287 = Unbundle By Name(w493) -> ("X"=w491:dbl, "Y"=w489:dbl)
                            n288 = Add(x=w497, y=w496) -> (x+y=w490:dbl)
                            n289 = Add(x=w494, y=w495) -> (x+y=w492:dbl)
                            n290 = Add(x=w490, y=w491) -> (x+y=w469:dbl)
                            n291 = Add(x=w489, y=w492) -> (x+y=w468:dbl)
                            n292 = local read "Use prediction"() -> (w471:bool)
                            n293 = case shown="True" w471 {
                              tunnel: w470 -> [w507 w509]
                              tunnel: w469 -> [w504 w511]
                              tunnel: w468 -> [w503 w512]
                              tunnel: [w505 w513] -> w465
                              tunnel: [w503 w512] -> w466
                              tunnel: [w504 w511] -> w467
                              frame False {
                                n294 = Unbundle By Name(w507) -> ("PRIORLib.IZOut"=w506:refnum<k7>)
                                n295 = call "IZGetPosition.vi"("PRIORLib.IZIn"=w506) -> ("ZPos"=w505:dbl)  [unwired: 1 in, 2 out]
                              }
                              frame True {
                                # "Use current Z as fallback"
                                n296 = local read "Minimum no. prediction points"() -> (w516:dbl)
                                n297 = Unbundle By Name(w509) -> ("focal map fileref"=w514:refnum<file>)
                                n298 = local read "Prediction order"() -> (w515:i16)
                                n299 = Unbundle By Name(w509) -> ("PRIORLib.IZOut"=w510:refnum<k7>)
                                n300 = call "IZGetPosition.vi"("PRIORLib.IZIn"=w510) -> ("ZPos"=w508:dbl)  [unwired: 1 in, 2 out]
                                n301 = call "predict_focus.vi"("focal map fileref"=w514, "Min prediction points"=w516, "Prediction order"=w515, "Known X"=w511, "Fallback Z"=w508, "Known Y"=w512) -> ("predicted focal position"=w513:dbl)  [unwired: 2 out]
                              }
                            }
                            n302 = local read "Well numbering mode"() -> (w486:u16)
                            n303 = case shown="1, Default" w486 {
                              tunnel: w476 -> [w520 w529]
                              tunnel: w474 -> [w519 w525]
                              tunnel: [w518 w527] -> w488
                              tunnel: [w517 w522] -> w487
                              frame 0 {
                                n304 = call "Build Text8"("Beginning Text"="", "Wi"=w520, "Wj"=w519) -> ("Result"=w518:string, "error out"=w517:errorcluster)  [unwired: 11 in]
                              }
                              frame 1, Default {
                                # "make well letter\nfrom number"
                                n305 = Add(x=65, y=w529) -> (x+y=w524:i32)
                                n306 = To Byte Integer(number=w524) -> (8bit integer=w523:i8)
                                n307 = Type Cast(x=w523) -> (*(type *) &x=w526:string)  [unwired: 1 in]
                                n308 = call "Build Text9"("Beginning Text"=w526, "well_j"=w525) -> ("Result"=w527:string, "error out"=w522:errorcluster)  [unwired: 12 in]
                              }
                            }
                            n309 = Bundle(w467, w466, "predicted focal position"=w465) -> (w481:T20)  [unwired: 1 in]
                            n310 = Unbundle By Name(w470) -> ("log fileref"=w485:refnum<file>)
                            n311 = call "Build Text7"("well"=w488, "Ni"=w473, "Nj"=w472, "error in (no error)"=w487) -> ("Result"=w482:string, "error out"=w484:errorcluster)  [unwired: 10 in]
                            n312 = Write to Text File(file (use dialog)=w485, text=w482, error in=w484) -> (error out=w483:errorcluster)  [unwired: 1 in, 2 out]
                            n313 = local write "error display"(w483) -> ()
                          }
                          frame #1 {
                            # "move"
                            n314 = Unbundle By Name(w538) -> ("PRIORLib.IScanOut"=w537:refnum<k7>)
                            n315 = Unbundle(w536) -> (w532:dbl, w531:dbl, "predicted focal position"=w530:dbl)
                            n316 = call "IScanMoveXYZAbs.vi"("PRIORLib.IScanIn"=w537, "XPos"=w532, "YPos"=w531, "ZPos"=w530) -> ("PRIORLib.IScanOut"=w535:refnum<k7>, "error out"=w534:errorcluster)  [unwired: 1 in, 1 out]
                            n317 = call "wait_for_movement.vi"("error in (no error)"=w534, "IScan in"=w535) -> ("error out"=w533:errorcluster)  [unwired: 8 in, 1 out]
                            n318 = local write "error display"(w533) -> ()
                          }
                          frame #2 {
                            # "open camera for focusing"
                            # "Reset camera ID"
                            # "Close camera"
                            # "autofocus"
                            n319 = local read "Camera settings"() -> (w555:T5)
                            n320 = call "start_camera_new.vi"("image type"=image_type."preview_image", "Camera settings"=w555) -> ("cameraId out"=w557:u32, "Refnum out"=w558:T7)  [unwired: 6 in, 2 out]
                            n321 = local read "Focus function"() -> (w545:u16)
                            n322 = local read "Prediction tolerance"() -> (w539:dbl)
                            n323 = Bundle By Name(cluster=w544, "Image Out"=w558, "cameraID"=w557) -> (w554:T9)
                            n324 = control-ref of="Preview"() -> (w542:refnum<vi>)
                            n325 = call "autofocus.vi"("dynamic scope variables"=w554, "Focus function"=w545, "Image display ref"=w542, "Prediction tolerance"=w539) -> ("dynamic scope variables out"=w549:T9, "Focus position"=w540:dbl, "Number of captures"=w541:i32)  [unwired: 1 in]
                            n326 = Bundle("Focus position"=w540, "Number of captures"=w541) -> (w543:T21)  [unwired: 1 in]
                            n327 = Unbundle By Name(w549) -> ("Image Out"=w551:T7, "cameraID"=w552:u32)
                            n328 = call <userlib>:"QCAM Grab Stop.vi"("cameraId"=w552) -> ("error out"=w547:errorcluster, "cameraId Out"=w553:u32)  [unwired: 1 in]
                            n329 = call <userlib>:"QCAM Close.vi"("error in (no error)"=w547, "cameraId"=w553) -> ("error out"=w548:errorcluster)  [unwired: 1 in]
                            n330 = call "IMAQ Dispose"("Image"=w551, "error in (no error)"=w548) -> ("error out"=w546:errorcluster)  [unwired: 4 in]
                            n331 = local write "error display"(w546) -> ()
                            n332 = Bundle By Name(cluster=w549, "cameraID"=u32 0) -> ()  [unwired: 1 out]
                          }
                          frame #3 {
                            # "go to most downward stack position"
                            n333 = Unbundle By Name(w568) -> ("PRIORLib.IScanOut"=w561:refnum<k7>, "PRIORLib.IZOut"=w562:refnum<k7>)
                            n334 = local read "No. of images in focal stack"() -> (w567:i32)
                            n335 = local read "Focal stack separation"() -> (w564:dbl)
                            n336 = Quotient & Remainder(x=w567, y=2) -> (floor(x/y)=w565:i32)  [unwired: 1 out]
                            n337 = Multiply(x=w565, y=w564) -> (x*y=w563:dbl)
                            n338 = call "IZMoveDown.vi"("Distance"=w563, "PRIORLib.IZIn"=w562) -> ("error out"=w560:errorcluster)  [unwired: 1 in, 2 out]
                            n339 = call "wait_for_movement.vi"("error in (no error)"=w560, "IScan in"=w561) -> ("error out"=w559:errorcluster)  [unwired: 8 in, 1 out]
                            n340 = local write "error display"(w559) -> ()
                          }
                          frame #4 {
                            # "Capture all images in focal stack"
                            n341 = local read "No. of images in focal stack"() -> (w588:i32)
                            n342 = local read "Camera settings"() -> (w585:T5)
                            n343 = local read "Well numbering mode"() -> (w580:u16)
                            n344 = Unbundle By Name(w570) -> ("Ni new"=w571:i32)
                            n345 = Unbundle By Name(w576) -> ("PRIORLib.IScanOut"=w575:refnum<k7>, "PRIORLib.IZOut"=w574:refnum<k7>)
                            n346 = Unbundle By Name(w570) -> ("Wi new"=w569:i32)
                            n347 = call "start_camera_new.vi"("image type"=image_type."capture_image", "Camera settings"=w585) -> ("cameraId out"=w579:u32, "Refnum out"=w578:T7)  [unwired: 6 in, 2 out]
                            n348 = for {
                              N: w588 -> [_]
                              tunnel: w571 -> [w605]
                              tunnel: w589 -> [w606]
                              tunnel: w569 -> [w610]
                              tunnel: w587 -> [w609]
                              tunnel: [w596] -> w581
                              tunnel: w580 -> [w608]
                              tunnel: w579 -> [w601]
                              tunnel: [w590] -> w577
                              tunnel: w575 -> [w592]
                              tunnel: w574 -> [w597]
                              shift-right: [w595] -> w573
                              shift-left: w578 -> [w600]
                              i -> [w607]
                              # "Handle numbering mode"
                              n349 = case shown="0" w608 {
                                tunnel: w610 -> [w617 w625]
                                tunnel: w609 -> [w616 w621]
                                tunnel: [w615 w623] -> w611
                                frame 0 {
                                n350 = call "Build Text2"("Beginning Text"="", "Wi"=w617, "Wj"=w616) -> ("Result"=w615:string)  [unwired: 11 in, 1 out]
                                }
                                frame 1, Default {
                                # "make well letter\nfrom number"
                                n351 = Add(x=65, y=w625) -> (x+y=w620:i32)
                                n352 = To Byte Integer(number=w620) -> (8bit integer=w619:i8)
                                n353 = Type Cast(x=w619) -> (*(type *) &x=w622:string)  [unwired: 1 in]
                                n354 = call "Build Text"("Beginning Text"=w622, "well_j"=w621) -> ("Result"=w623:string)  [unwired: 12 in, 1 out]
                                }
                              }
                              n355 = local read "File name base"() -> (w613:string)
                              n356 = local read "Image Output directory"() -> (w604:path)
                              n357 = call "Build Text"("Beginning Text"=w613, "Nk"=w607, "well"=w611, "Ni"=w605, "Nj"=w606) -> ("Result"=w612:string, "error out"=w603:errorcluster)  [unwired: 9 in]
                              n358 = Build Path(base path=w604, name or relative path=w612) -> (appended path=w602:path)
                              n359 = call <userlib>:"QCAM Grab Acquire.vi"("error in (no error)"=w603, "Image"=w600, "cameraId"=w601) -> ("error out"=w593:errorcluster, "Image Out"=w594:T7, "cameraId out"=w596:u32)
                              n360 = call-poly "IMAQ Write File 2"("error in (no error)"=w593, "File Path"=w602, "Image"=w594) -> ("error out"=w598:errorcluster, "Image Out (duplicate)"=w595:T7)  [unwired: 7 in]
                              n361 = local read "Focal stack separation"() -> (w599:dbl)
                              n362 = call "IMAQ Histograph"("Image"=w595) -> ("Histogram Graph"=w614:T6)  [unwired: 7 in, 3 out]
                              n363 = local write "Preview"(w595) -> ()
                              n364 = local write "Histogram"(w614) -> ()
                              n365 = call "IZMoveUp.vi"("Distance"=w599, "error in (no error)"=w598, "PRIORLib.IZIn"=w597) -> ("error out"=w591:errorcluster)  [unwired: 2 out]
                              n366 = call "wait_for_movement.vi"("error in (no error)"=w591, "IScan in"=w592) -> ("error out"=w590:errorcluster)  [unwired: 8 in, 1 out]
                            }
                            n367 = call <userlib>:"QCAM Grab Stop.vi"("error in (no error)"=w577, "cameraId"=w581) -> ("error out"=w583:errorcluster, "cameraId Out"=w584:u32)
                            n368 = call <userlib>:"QCAM Close.vi"("error in (no error)"=w583, "cameraId"=w584) -> ("error out"=w582:errorcluster)  [unwired: 1 in]
                            n369 = call "IMAQ Dispose"("Image"=w573, "error in (no error)"=w582) -> ("error out"=w572:errorcluster)  [unwired: 4 in]
                            n370 = local write "error display"(w572) -> ()
                          }
                          frame #5 {
                            # "Set pixel on scan map"
                            n371 = Unbundle By Name(w628) -> ("Wi new"=w626:i32, "Ni new"=w627:i32)
                            n372 = local read "Movement controls"() -> (w637:T2)
                            n373 = Unbundle By Name(w637) -> ("Nx"=w636:i32, "Ny"=w635:i32)
                            n374 = formula code="int32 x;\nint32 y;\n\nx = (Wi*(nx+1)) +ni;\ny = (Wj*(ny+1)) +nj;"("nx"=w636, "ny"=w635, "Wi"=w626, "Wj"=w630, "ni"=w627, "nj"=w629) -> ("x"=w639:i32, "y"=w640:i32)
                            n375 = Unbundle By Name(w634) -> ("Scan map"=w633:T7)
                            n376 = call "IMAQ SetPixelValue"("Pixel Value"=u8 255, "Y Coordinate"=w640, "X Coordinate"=w639, "Image"=w633) -> ("error out"=w631:errorcluster, "Image Out"=w632:T7)  [unwired: 6 in]
                            n377 = local write "Scan map viewer"(w632) -> ()
                            n378 = local write "error display"(w631) -> ()
                          }
                          frame #6 {
                            # "Handle case that no cells are present"
                            # "return to original focus position"
                            n379 = Unbundle By Name(w646) -> ("PRIORLib.IScanOut"=w644:refnum<k7>, "PRIORLib.IZOut"=w645:refnum<k7>)
                            n380 = Unbundle(w643) -> ("Focus position"=w641:dbl)  [unwired: 1 out]
                            n381 = Not A Number/Path/Refnum?(number/path/refnum=w641) -> (NaN/Path/Refnum?=w642:bool)
                            n382 = case shown="False" w642 {
                              tunnel: w645 -> [w651 _]
                              tunnel: w644 -> [w650 _]
                              tunnel: w641 -> [w647 _]
                              frame False {
                                n383 = call "IZMoveAbs.vi"("Location"=w647, "PRIORLib.IZIn"=w651) -> ("error out"=w649:errorcluster)  [unwired: 1 in, 2 out]
                                n384 = call "wait_for_movement.vi"("error in (no error)"=w649, "IScan in"=w650) -> ("error out"=w648:errorcluster)  [unwired: 8 in, 1 out]
                                n385 = local write "error display"(w648) -> ()
                              }
                              frame True {
                              }
                            }
                          }
                          frame #7 {
                            # "Wi, Wj, Ni, Nj, absX, absY, Z, no. of captures, prediction"
                            # "Save focus postion to focal map file"
                            # "If emergency stop, close application to avoid moving back to the origin"
                            n386 = Unbundle By Name(w660) -> ("focal map fileref"=w667:refnum<file>)
                            n387 = Unbundle By Name(w657) -> ("Wi new"=w656:i32, "Ni new"=w655:i32)
                            n388 = Unbundle(w668) -> (w653:dbl, w652:dbl, "predicted focal position"=w654:dbl)
                            n389 = Unbundle(w663) -> ("Focus position"=w662:dbl, "Number of captures"=w661:i32)
                            n390 = Format Into String(format string="%d,%d,%d,%d,%f,%f,%f,%d,%f\\n", initial string=w667, w656, w665, w655, w664, w653, w652, w662, w661, w654) -> (error out=w659:errorcluster)  [unwired: 1 in, 1 out]
                            n391 = local write "error display"(w659) -> ()
                            n392 = global read "Globals.vi" "EmerStop"() -> (w658:bool)
                            n393 = Stop(stop? (T)=w658) -> ()
                          }
                        }
                      }
                      frame True {
                      }
                    }
                  }
                }
              }
            }
          }
          frame 1 {
            n394 = local read "Focus file path"() -> (w677:path)
            n395 = call-poly <vilib>:"Read From Spreadsheet File.vi"("delimiter (\\t)"="," ("delimiter (\\t)"), "file path (dialog if empty)"=w677) -> ("first row"=w671:dbl[], "all rows"=w670:dbl[][])  [unwired: 5 in, 3 out]
            n396 = call "remove_csv_header.vi"("first row"=w671, "all rows"=w670) -> ("array w/ subset deleted"=w669:dbl[][])  [unwired: 1 out]
            n397 = Array Size(array=w669) -> (size(s)=w675:i32[])
            n398 = Index Array(array=w675, index=0) -> (element=w673:i32)
            n399 = for {
              N: w673 -> [_]
              tunnel: w669 -> [w703] mode=indexing
              tunnel: w672 -> [w697]
              stop <- w692 continue-if-true
              # "Nj"
              # "Ni"
              # "Wj"
              # "Wi"
              # "Z"
              # "Y"
              # "X"
              n400 = Unbundle By Name(w697) -> ("PRIORLib.IScanOut"=w718:refnum<k7>, "PRIORLib.IZOut"=w689:refnum<k7>)
              n401 = Index Array(array=w703, index=4) -> (element=w682:dbl)
              n402 = Index Array(array=w703, index=5) -> (element=w684:dbl)
              n403 = Index Array(array=w703, index=6) -> (element=w678:dbl)
              n404 = Index Array(array=w703, index=2) -> (element=w704:dbl)
              n405 = Index Array(array=w703, index=3) -> (element=w705:dbl)
              n406 = Index Array(array=w703, index=0) -> (element=w724:dbl)
              n407 = Index Array(array=w703, index=1) -> (element=w723:dbl)
              n408 = To Unsigned Long Integer(number=w704) -> (unsigned 32bit integer=w700:u32)
              n409 = To Unsigned Long Integer(number=w724) -> (unsigned 32bit integer=w702:u32)
              n410 = To Unsigned Long Integer(number=w705) -> (unsigned 32bit integer=w699:u32)
              n411 = To Unsigned Long Integer(number=w723) -> (unsigned 32bit integer=w701:u32)
              n412 = local read "Focus offset"() -> (w679:dbl)
              n413 = local read "Y offset"() -> (w680:dbl)
              n414 = local read "X offset"() -> (w681:dbl)
              n415 = local read "No. of images in focal stack"() -> (w733:i32)
              n416 = Add(x=w679, y=w678) -> (x+y=w687:dbl)
              n417 = Add(x=w680, y=w684) -> (x+y=w685:dbl)
              n418 = Add(x=w681, y=w682) -> (x+y=w683:dbl)
              n419 = local read "Movement controls"() -> (w710:T2)
              n420 = local read "Focal stack separation"() -> (w734:dbl)
              n421 = call "IScanMoveXYZAbs.vi"("PRIORLib.IScanIn"=w718, "XPos"=w683, "YPos"=w685, "ZPos"=w687) -> ("PRIORLib.IScanOut"=w688:refnum<k7>, "error out"=w686:errorcluster)  [unwired: 1 in, 1 out]
              n422 = Unbundle By Name(w710) -> ("Nx"=w709:i32, "Ny"=w708:i32)
              n423 = call "wait_for_movement.vi"("error in (no error)"=w686, "IScan in"=w688) -> ("error out"=w732:errorcluster, "IScan out"=w735:refnum<k7>)  [unwired: 8 in]
              n424 = Quotient & Remainder(x=w733, y=2) -> (floor(x/y)=w737:i32)  [unwired: 1 out]
              n425 = formula code="int32 x;\nint32 y;\n\nx = (Wi*(nx+1)) +ni;\ny = (Wj*(ny+1)) +nj;"("nx"=w709, "ny"=w708, "Wi"=w702, "Wj"=w701, "ni"=w700, "nj"=w699) -> ("x"=w695:i32, "y"=w694:i32)
              n426 = Multiply(x=w737, y=w734) -> (x*y=w691:dbl)
              n427 = Unbundle By Name(w697) -> ("Scan map"=w696:T7)
              n428 = call "IZMoveDown.vi"("Distance"=w691, "error in (no error)"=w732, "PRIORLib.IZIn"=w689) -> ("error out"=w736:errorcluster, "PRIORLib.IZOut"=w719:refnum<k7>)  [unwired: 1 out]
              n429 = local read "No. of images in focal stack"() -> (w728:i32)
              n430 = local read "Camera settings"() -> (w731:T5)
              n431 = local read "Well numbering mode"() -> (w725:u16)
              n432 = call "wait_for_movement.vi"("error in (no error)"=w736, "IScan in"=w735) -> ("error out"=w729:errorcluster, "IScan out"=w720:refnum<k7>)  [unwired: 8 in]
              n433 = call "IMAQ SetPixelValue"("Pixel Value"=u8 255, "Y Coordinate"=w694, "X Coordinate"=w695, "Image"=w696) -> ("Image Out"=w693:T7)  [unwired: 6 in, 1 out]
              n434 = local write "Scan map viewer"(w693) -> ()
              n435 = call "start_camera_new.vi"("error in (no error)"=w729, "image type"=image_type."capture_image", "Camera settings"=w731) -> ("error out"=w711:errorcluster, "cameraId out"=w722:u32, "Refnum out"=w721:T7)  [unwired: 5 in, 1 out]
              n436 = for {
                N: w728 -> [_]
                tunnel: w725 -> [w767]
                tunnel: w702 -> [w766]
                tunnel: w701 -> [w765]
                tunnel: w722 -> [w756]
                tunnel: w720 -> [w752]
                tunnel: w719 -> [w751]
                shift-right: [w749] -> w712
                shift-left: w721 -> [w755]
                tunnel: [w748] -> w714
                tunnel: [w747] -> w713
                tunnel: w711 -> [w746]
                tunnel: w700 -> [w744]
                tunnel: w699 -> [w743]
                i -> [w745]
                n437 = case shown="0" w767 {
                  tunnel: w766 -> [w770 w778]
                  tunnel: w765 -> [w769 w774]
                  tunnel: [w768 w776] -> w759
                  frame 0 {
                    n438 = call "Build Text3"("Beginning Text"="", "Wi"=w770, "Wj"=w769) -> ("Result"=w768:string)  [unwired: 11 in, 1 out]
                  }
                  frame 1, Default {
                    # "make well letter\nfrom number"
                    n439 = Add(x=65, y=w778) -> (x+y=w773:u32)
                    n440 = To Byte Integer(number=w773) -> (8bit integer=w772:i8)
                    n441 = Type Cast(x=w772) -> (*(type *) &x=w775:string)  [unwired: 1 in]
                    n442 = call "Build Text4"("Beginning Text"=w775, "well_j"=w774) -> ("Result"=w776:string)  [unwired: 12 in, 1 out]
                  }
                }
                n443 = local read "File name base"() -> (w757:string)
                n444 = local read "Image Output directory"() -> (w758:path)
                n445 = call "Build Text5"("Beginning Text"=w757, "Nk"=w745, "well"=w759, "Ni"=w744, "Nj"=w743, "error in (no error)"=w746) -> ("Result"=w764:string, "error out"=w763:errorcluster)  [unwired: 8 in]
                n446 = Build Path(base path=w758, name or relative path=w764) -> (appended path=w762:path)
                n447 = call <userlib>:"QCAM Grab Acquire.vi"("error in (no error)"=w763, "Image"=w755, "cameraId"=w756) -> ("error out"=w760:errorcluster, "Image Out"=w761:T7, "cameraId out"=w748:u32)
                n448 = local read "Focal stack separation"() -> (w742:dbl)
                n449 = call-poly "IMAQ Write File 2"("error in (no error)"=w760, "File Path"=w762, "Image"=w761) -> ("error out"=w753:errorcluster, "Image Out (duplicate)"=w749:T7)  [unwired: 7 in]
                n450 = call "IMAQ Histograph"("Image"=w749) -> ("Histogram Graph"=w750:T6)  [unwired: 7 in, 3 out]
                n451 = local write "Preview"(w749) -> ()
                n452 = call "IZMoveUp.vi"("Distance"=w742, "error in (no error)"=w753, "PRIORLib.IZIn"=w751) -> ("error out"=w754:errorcluster)  [unwired: 2 out]
                n453 = local write "Histogram"(w750) -> ()
                n454 = call "wait_for_movement.vi"("error in (no error)"=w754, "IScan in"=w752) -> ("error out"=w747:errorcluster)  [unwired: 8 in, 1 out]
              }
              n455 = call <userlib>:"QCAM Grab Stop.vi"("error in (no error)"=w713, "cameraId"=w714) -> ("error out"=w716:errorcluster, "cameraId Out"=w717:u32)
              n456 = local read "Run test button"() -> (w692:bool)
              n457 = call <userlib>:"QCAM Close.vi"("error in (no error)"=w716, "cameraId"=w717) -> ("error out"=w715:errorcluster)  [unwired: 1 in]
              n458 = call "IMAQ Dispose"("Image"=w712, "error in (no error)"=w715) -> ("error out"=w690:errorcluster)  [unwired: 4 in]
              n459 = local write "error display"(w690) -> ()
            }
          }
        }
      }
      frame "Test clean" {
        # "Send email to mark completion"
        # "Close log file"
        # "Return to origin"
        # "Rescale histogram for 8-bit pixels"
        # "Reset camera ID"
        # "Reset button"
        # "Make controls active again"
        n460 = stacked-sequence {
          tunnel: T10."Enabled" ("Disabled") -> [w812 w813 w814 w815 w816 w817 w818 w819 w820]
          frame #0 {
            n461 = property on="Movement controls" class="Clust (strict)"("DisabledEnum"=w812) -> ()  [unwired: 2 in, 2 out]
          }
          frame #1 {
            n462 = property on="Preset controls" class="Clust (strict)"("DisabledEnum"=w813) -> ()  [unwired: 2 in, 2 out]
          }
          frame #2 {
            n463 = property on="Camera settings" class="Clust (strict)"("DisabledEnum"=w814) -> ()  [unwired: 2 in, 2 out]
          }
          frame #3 {
            n464 = property on="File name base" class="Str"("DisabledEnum"=w815) -> ()  [unwired: 2 in, 2 out]
          }
          frame #4 {
            n465 = property on="Image Output directory" class="Path"("DisabledEnum"=w816) -> ()  [unwired: 2 in, 2 out]
          }
          frame #5 {
            n466 = property on="Origin controls" class="Clust (strict)"("DisabledEnum"=w817) -> ()  [unwired: 2 in, 2 out]
          }
          frame #6 {
            n467 = property on="Single step controls" class="Clust (strict)"("DisabledEnum"=w818) -> ()  [unwired: 2 in, 2 out]
          }
          frame #7 {
            n468 = property on="camera button" class="Bool (strict)"("DisabledEnum"=w819) -> ()  [unwired: 2 in, 2 out]
          }
          frame #8 {
            n469 = property on="close button" class="Bool (strict)"("DisabledEnum"=w820) -> ()  [unwired: 2 in, 2 out]
          }
        }
        n470 = local read "Focus mode"() -> (w791:u16)
        n471 = case shown="0, Default" w791 {
          tunnel: w790 -> [w811 _]
          frame 0, Default {
            # "Close focal map file"
            n472 = Unbundle By Name(w811) -> ("focal map fileref"=w810:refnum<file>)
            n473 = Close File(refnum=w810) -> ()  [unwired: 1 in, 2 out]
          }
          frame 1 {
          }
        }
        n474 = local read "Origin controls"() -> (w795:T3)
        n475 = Unbundle By Name(w790) -> ("PRIORLib.IScanOut"=w792:refnum<k7>)
        n476 = Unbundle By Name(w795) -> ("X"=w794:dbl, "Y"=w793:dbl)
        n477 = local write "Run test button"(FALSE ("Run test button")) -> ()
        n478 = call "IScanMoveXYZAbs.vi"("PRIORLib.IScanIn"=w792, "XPos"=w794, "YPos"=w793, "ZPos"=0.0, "error in (no error)"=w788) -> ("error out"=w787:errorcluster)  [unwired: 2 out]
        n479 = local read "Completion email address"() -> (w784:string)
        n480 = Bundle By Name(cluster=w790, "cameraID"=u32 0) -> (w782:T9)
        n481 = Not Equal?(x="", y=w784) -> (x != y?=w786:bool)
        n482 = property on="Histogram" class="WFGraph (strict)"("XScale.Maximum"=255.0 ("X Scale.Range:Maximum")) -> ()  [unwired: 2 in, 2 out]
        n483 = Unbundle By Name(w782) -> ("log fileref"=w781:refnum<file>)
        n484 = Refnum to Path(1:w781) -> (0:w780:path)
        n485 = case shown="True" w786 {
          tunnel: w787 -> [w803 w808]
          tunnel: w780 -> [_ _]
          tunnel: [w803 w805] -> w779
          tunnel: w784 -> [_ w804]
          frame False {
          }
          frame True {
            n486 = local read "File name base"() -> (w809:string)
            n487 = call "email text"("batch name"=w809, "error in (no error)"=w808) -> ("Result"=w807:string, "error out"=w806:errorcluster)  [unwired: 12 in]
            n488 = call "email.vi"("error in (no error)"=w806, "Body"=w807, "Recipient's Email Address Address"=w804) -> ("error out"=w805:errorcluster)  [unwired: 1 in]
          }
        }
        n489 = Close File(refnum=w781, error in=w779) -> (error out=w783:errorcluster)  [unwired: 1 out]
        n490 = call "Display Message to User"("error in (no error)"=w783) -> ("error out"=w789:errorcluster)  [unwired: 9 in, 1 out]
      }
      frame "Close" {
        # "Close camera connection"
        # "Turn off connection indicator"
        # "Set buttons to off"
        # "Close connections to stage"
        n491 = Unbundle By Name(w824) -> ("PRIORLib.IScanOut"=w827:refnum<k7>, "PRIORLib.IStageOut"=w828:refnum<k7>, "PRIORLib.IFilterOut"=w830:refnum<k7>, "PRIORLib.IZOut"=w829:refnum<k7>)
        n492 = stacked-sequence {
          tunnel: w824 -> [w838]
          tunnel: [w834] -> w821
          tunnel: w822 -> [w833]
          frame #0 {
            n493 = Unbundle By Name(w838) -> ("cameraID"=w836:u32, "Image Out"=w835:T7)
            n494 = Not Equal To 0?(x=w836) -> (x != 0?=w837:bool)
            n495 = case shown="False" w837 {
              tunnel: w836 -> [_ w844]
              tunnel: w835 -> [_ w843]
              tunnel: [w839 w841] -> w834
              tunnel: w833 -> [w839 w840]
              frame False {
              }
              frame True {
                n496 = call <userlib>:"QCAM Grab Stop.vi"("error in (no error)"=w840, "cameraId"=w844) -> ("error out"=w845:errorcluster, "cameraId Out"=w846:u32)
                n497 = call <userlib>:"QCAM Close.vi"("error in (no error)"=w845, "cameraId"=w846) -> ("error out"=w842:errorcluster)  [unwired: 1 in]
                n498 = call "IMAQ Dispose"("Image"=w843, "error in (no error)"=w842) -> ("error out"=w841:errorcluster)  [unwired: 4 in]
              }
            }
          }
        }
        n499 = stacked-sequence {
          tunnel: w827 -> [_ _ _ w858]
          tunnel: w828 -> [_ _ w857 _]
          tunnel: w830 -> [w855 _ _ _]
          tunnel: w829 -> [_ w856 _ _]
          frame #0 {
            n500 = call "IFilterClose.vi"("PRIORLib.IFilter"=w855) -> ()  [unwired: 1 out]
          }
          frame #1 {
            n501 = call "IZClose.vi"("PRIORLib.IZ"=w856) -> ()  [unwired: 1 out]
          }
          frame #2 {
            n502 = call "IStageClose.vi"("PRIORLib.IStage"=w857) -> ()  [unwired: 1 out]
          }
          frame #3 {
            n503 = call "IScanClose.vi"("PRIORLib.IScan"=w858) -> ()  [unwired: 2 out]
          }
        }
        n504 = stacked-sequence {
          tunnel: FALSE ("Value") -> [w847 w848 w849 w850 w851 w852 w853]
          frame #0 {
            n505 = property on="auto expose button" class="Bool (strict)"("Value"=w847) -> ()  [unwired: 2 in, 2 out]
          }
          frame #1 {
            n506 = property on="set origin button" class="Bool (strict)"("Value"=w848) -> ()  [unwired: 2 in, 2 out]
          }
          frame #2 {
            n507 = property on="save preset button" class="Bool (strict)"("Value"=w849) -> ()  [unwired: 2 in, 2 out]
          }
          frame #3 {
            n508 = property on="Run test button" class="Bool (strict)"("Value"=w850) -> ()  [unwired: 2 in, 2 out]
          }
          frame #4 {
            n509 = property on="close button" class="Bool (strict)"("Value"=w851) -> ()  [unwired: 2 in, 2 out]
          }
          frame #5 {
            n510 = property on="camera button" class="Bool (strict)"("Value"=w852) -> ()  [unwired: 2 in, 2 out]
          }
          frame #6 {
            n511 = Bundle("Value"=w853, "Value"=w853, "Value"=w853, "Value"=w853, "Value"=w853) -> (w854:T15)  [unwired: 1 in]
            n512 = property on="Single step controls" class="Clust (strict)"("Value"=w854) -> ()  [unwired: 2 in, 2 out]
          }
        }
        n513 = local write "connection indicator"(FALSE ("connection indicator")) -> ()
      }
    }
    n514 = Wait (ms)(milliseconds to wait=u32 50) -> ()  [unwired: 1 out]
    n515 = local write "error display"(w3) -> ()
    n516 = call "log_errors.vi"("error in (no error)"=w3, "dynamic data"=w4) -> ()  [unwired: 1 in]
  }
  n517 = while {
    i -> [w859]
    stop <- w861 stop-if-true
    n518 = event shown="[2] \"emergency stop\": Value Change" {
      selector: _ -> [_ _ _]
      dyn-events: _ -> [_ _ _]
      timeout: 25 -> [_ _ _]
      tunnel: w859 -> [w867 _ _]
      event Timeout {
        # "Display time if not emergency stop"
        n519 = event-data() -> ()  [unwired: 1 in, 2 out]
        n520 = local read "Run test button"() -> (w863:bool)
        n521 = Quotient & Remainder(x=w867, y=40) -> (x-y*floor(x/y)=w865:i32)  [unwired: 1 out]
        n522 = Equal To 0?(x=w865) -> (x = 0?=w864:bool)
        n523 = And(x=w863, y=w864) -> (x .and. y?=w862:bool)
        n524 = case shown="True" w862 {
          frame False {
          }
          frame True {
            n525 = local read "Scan map viewer"() -> (w868:T7)
            n526 = Tick Count (ms)() -> (millisecond timer value=w872:u32)
            n527 = call "time_display.vi"("scan map in"=w868, "test start time"="test start time", "millisecond timer value"=w872) -> ("estimated time remaining"=→"estimated remaining":string, "elapsed time"=→"elapsed time":string)  [unwired: 7 in]
          }
        }
      }
      event Key Down {
        n528 = event-data() -> ("VKey"=w875:T22)  [unwired: 1 in, 5 out]
        n529 = Equal?(x=eventvkey."Escape", y=w875) -> (x = y?=w873:bool)
        n530 = case shown="True" w873 {
          frame False {
          }
          frame True {
            w876 = TRUE
            n531 = call "Display Message to User3"() -> ()  [unwired: 10 in, 2 out]
            n532 = global write "Globals.vi" "EmerStop"(w876) -> ()
            n533 = global write "QCam Grab Abort.vi" "Grab Abort"(w876) -> ()
          }
        }
      }
      event "emergency stop": Value Change {
        n534 = event-data() -> ("NewVal"=w877:bool)  [unwired: 1 in, 4 out]
        n535 = case shown="True" w877 {
          frame False {
          }
          frame True {
            w878 = TRUE
            n536 = call "Display Message to User2"() -> ()  [unwired: 10 in, 2 out]
            n537 = global write "Globals.vi" "EmerStop"(w878) -> ()
            n538 = global write "QCam Grab Abort.vi" "Grab Abort"(w878) -> ()
          }
        }
      }
    }
    n539 = local read "close button"() -> (w861:bool)
  }
